vi "lv_icon.vi"(10 "Color icon in":T4={"image type"=0, "image depth"=8, "image"=[255, 255, 255, 255, 255, 255, 255, 255, 255, 255, 255, 255, 255, 255, 255, 255, 255, 255, 255, 255, 255, 255, 255, 255, 255, 255, 255, 255, 255, 255, 255, 255, 255, 0, 0, 0, 0, 0, 0, 0, 0, 0, 0, 0, 0, 0, 0, 0, 0, 0, 0, 0, 0, 0, 0, 0, 0, 0, 0, 0, 0, 0, 0, 255, 255, 0, 0, 0, 0, 0, 0, 0, 0, 0, 0, 0, 0, 0, 0, 0, 0, 0, 0, 0, 0, 0, 0, 0, 0, 0, 0, 0, 0, 0, 0, 255, 255, 0, 0, 255, 255, 255, 255, 255, 255, 255, 255, 255, 255, 255, 255, 255, 255, 255, 255, 255, 255, 255, 0, 0, 0, 0, 0, 0, 0, 0, 0, 255, 255, 0, 0, 255, 250, 250, 250, 250, 250, 250, 250, 250, 250, 250, 250, 250, 248, 250, 44, 250, 44, 255, 0, 0, 0, 0, 0, 0, 0, 0, 0, 255, 255, 0, 0, 255, 250, 255, 255, 255, 255, 255, 255, 255, 255, 255, 255, 255, 248, 250, 44, 250, 44, 255, 0, 0, 0, 0, 0, 0, 0, 0, 0, 255, 255, 0, 0, 255, 250, 255, 209, 197, 209, 255, 255, 255, 209, 197, 209, 255, 248, 252, 43, 252, 44, 255, 0, 0, 0, 0, 0, 0, 0, 0, 0, 255, 255, 0, 0, 255, 250, 255, 197, 255, 197, 255, 255, 255, 197, 255, 197, 255, 248, 44, 44, 44, 44, 255, 0, 0, 0, 0, 0, 0, 0, 0, 0, 255, 255, 0, 0, 255, 250, 209, 197, 255, 197, 209, 255, 209, 197, 255, 197, 209, 248, 43, 252, 43, 44, 255, 0, 0, 0, 0, 0, 0, 0, 0, 0, 255, 255, 0, 0, 255, 250, 197, 209, 255, 209, 197, 255, 197, 209, 255, 209, 197, 248, 252, 8, 252, 44, 255, 0, 0, 0, 0, 0, 0, 0, 0, 0, 255, 255, 0, 0, 255, 250, 197, 255, 255, 255, 197, 255, 197, 255, 255, 255, 197, 248, 252, 8, 252, 44, 255, 0, 0, 0, 0, 0, 0, 0, 0, 0, 255, 255, 0, 0, 255, 250, 255, 255, 255, 255, 209, 197, 209, 255, 255, 255, 255, 248, 43, 252, 43, 44, 255, 0, 0, 0, 0, 0, 0, 0, 0, 0, 255, 255, 0, 0, 255, 250, 255, 255, 255, 255, 255, 255, 255, 255, 255, 255, 255, 248, 44, 44, 44, 44, 255, 0, 0, 0, 0, 0, 0, 0, 0, 0, 255, 255, 0, 0, 255, 248, 248, 248, 248, 248, 248, 248, 248, 248, 248, 248, 248, 248, 44, 44, 131, 131, 255, 0, 0, 0, 0, 0, 0, 0, 0, 0, 255, 255, 0, 0, 255, 44, 44, 44, 44, 44, 44, 44, 44, 44, 44, 44, 44, 44, 44, 44, 131, 5, 131, 131, 0, 0, 0, 0, 0, 0, 0, 0, 255, 255, 0, 0, 255, 44, 252, 44, 44, 44, 44, 44, 252, 44, 44, 44, 44, 35, 35, 35, 131, 5, 5, 5, 131, 131, 0, 0, 0, 0, 0, 0, 255, 255, 0, 0, 255, 252, 213, 252, 44, 44, 44, 252, 35, 252, 44, 35, 35, 44, 44, 44, 131, 5, 5, 255, 5, 5, 131, 131, 0, 0, 0, 0, 255, 255, 0, 0, 255, 44, 212, 44, 44, 44, 44, 35, 44, 44, 35, 44, 44, 44, 44, 44, 131, 5, 255, 255, 255, 5, 5, 5, 131, 35, 35, 0, 255, 255, 0, 0, 255, 255, 213, 255, 255, 255, 35, 255, 255, 35, 255, 255, 255, 255, 255, 255, 131, 5, 5, 255, 5, 5, 131, 131, 0, 0, 0, 0, 255, 255, 0, 0, 0, 0, 212, 0, 0, 0, 35, 0, 0, 35, 0, 0, 213, 212, 212, 213, 131, 5, 5, 5, 131, 131, 0, 0, 0, 0, 0, 0, 255, 255, 0, 0, 0, 0, 0, 213, 0, 0, 0, 35, 35, 0, 0, 212, 0, 0, 0, 0, 131, 5, 131, 131, 0, 0, 0, 0, 0, 0, 0, 0, 255, 255, 0, 0, 0, 0, 0, 0, 212, 212, 0, 0, 0, 0, 213, 0, 0, 0, 0, 0, 131, 131, 0, 0, 0, 0, 0, 0, 0, 0, 0, 0, 255, 255, 0, 0, 0, 0, 0, 0, 0, 0, 213, 212, 213, 212, 0, 0, 0, 0, 0, 0, 0, 0, 0, 0, 0, 0, 255, 255, 0, 0, 0, 0, 255, 255, 0, 0, 0, 0, 0, 0, 0, 0, 0, 0, 0, 0, 0, 0, 0, 0, 0, 0, 0, 0, 0, 0, 0, 255, 0, 0, 255, 0, 0, 0, 255, 255, 0, 0, 0, 0, 0, 0, 0, 0, 0, 0, 0, 0, 0, 0, 0, 0, 0, 0, 0, 0, 0, 0, 0, 0, 0, 0, 255, 0, 0, 0, 255, 255, 0, 0, 0, 0, 0, 0, 0, 0, 0, 0, 0, 0, 0, 0, 0, 0, 0, 0, 0, 0, 0, 0, 0, 0, 255, 255, 0, 0, 0, 0, 255, 255, 0, 0, 0, 0, 0, 0, 0, 0, 0, 0, 0, 0, 0, 0, 0, 0, 0, 0, 0, 0, 0, 0, 0, 0, 0, 0, 255, 0, 0, 0, 255, 255, 0, 0, 0, 0, 0, 0, 0, 0, 0, 0, 0, 0, 0, 0, 0, 0, 0, 0, 0, 0, 0, 0, 0, 255, 0, 0, 255, 0, 0, 0, 255, 255, 0, 0, 0, 0, 0, 0, 0, 0, 0, 0, 0, 0, 0, 0, 0, 0, 0, 0, 0, 0, 0, 0, 0, 0, 255, 255, 0, 0, 0, 0, 255, 255, 0, 0, 0, 0, 0, 0, 0, 0, 0, 0, 0, 0, 0, 0, 0, 0, 0, 0, 0, 0, 0, 0, 0, 0, 0, 0, 0, 0, 0, 0, 255, 255, 0, 0, 0, 0, 0, 0, 0, 0, 0, 0, 0, 0, 0, 0, 0, 0, 0, 0, 0, 0, 0, 0, 0, 0, 0, 0, 0, 0, 0, 0, 255, 255, 255, 255, 255, 255, 255, 255, 255, 255, 255, 255, 255, 255, 255, 255, 255, 255, 255, 255, 255, 255, 255, 255, 255, 255, 255, 255, 255, 255, 255, 255, 255], "mask"=[], "colors"=[16777215, 16777164, 16777113, 16777062, 16777011, 16776960, 16764159, 16764108, 16764057, 16764006, 16763955, 16763904, 16751103, 16751052, 16751001, 16750950, 16750899, 16750848, 16738047, 16737996, 16737945, 16737894, 16737843, 16737792, 16724991, 16724940, 16724889, 16724838, 16724787, 16724736, 16711935, 16711884, 16711833, 16711782, 16711731, 16711680, 13434879, 13434828, 13434777, 13434726, 13434675, 13434624, 13421823, 13421772, 13421721, 13421670, 13421619, 13421568, 13408767, 13408716, 13408665, 13408614, 13408563, 13408512, 13395711, 13395660, 13395609, 13395558, 13395507, 13395456, 13382655, 13382604, 13382553, 13382502, 13382451, 13382400, 13369599, 13369548, 13369497, 13369446, 13369395, 13369344, 10092543, 10092492, 10092441, 10092390, 10092339, 10092288, 10079487, 10079436, 10079385, 10079334, 10079283, 10079232, 10066431, 10066380, 10066329, 10066278, 10066227, 10066176, 10053375, 10053324, 10053273, 10053222, 10053171, 10053120, 10040319, 10040268, 10040217, 10040166, 10040115, 10040064, 10027263, 10027212, 10027161, 10027110, 10027059, 10027008, 6750207, 6750156, 6750105, 6750054, 6750003, 6749952, 6737151, 6737100, 6737049, 6736998, 6736947, 6736896, 6724095, 6724044, 6723993, 6723942, 6723891, 6723840, 6711039, 6710988, 6710937, 6710886, 6710835, 6710784, 6697983, 6697932, 6697881, 6697830, 6697779, 6697728, 6684927, 6684876, 6684825, 6684774, 6684723, 6684672, 3407871, 3407820, 3407769, 3407718, 3407667, 3407616, 3394815, 3394764, 3394713, 3394662, 3394611, 3394560, 3381759, 3381708, 3381657, 3381606, 3381555, 3381504, 3368703, 3368652, 3368601, 3368550, 3368499, 3368448, 3355647, 3355596, 3355545, 3355494, 3355443, 3355392, 3342591, 3342540, 3342489, 3342438, 3342387, 3342336, 65535, 65484, 65433, 65382, 65331, 65280, 52479, 52428, 52377, 52326, 52275, 52224, 39423, 39372, 39321, 39270, 39219, 39168, 26367, 26316, 26265, 26214, 26163, 26112, 13311, 13260, 13209, 13158, 13107, 13056, 255, 204, 153, 102, 51, 15597568, 14483456, 12255232, 11141120, 8912896, 7798784, 5570560, 4456448, 2228224, 1114112, 60928, 56576, 47872, 43520, 34816, 30464, 21760, 17408, 8704, 4352, 238, 221, 187, 170, 136, 119, 85, 68, 34, 17, 15658734, 14540253, 12303291, 11184810, 8947848, 7829367, 5592405, 4473924, 2236962, 1118481, 0], "Rectangle"={"left"=0, "top"=0, "right"=32, "bottom"=32}}, 11 "BW icon in":T4={"image type"=0, "image depth"=1, "image"=[255, 255, 255, 255, 128, 0, 0, 1, 128, 0, 0, 1, 159, 255, 252, 1, 144, 0, 84, 1, 151, 255, 84, 1, 150, 251, 84, 1, 149, 117, 4, 1, 149, 117, 36, 1, 147, 174, 84, 1, 147, 174, 84, 1, 151, 223, 36, 1, 151, 255, 4, 1, 144, 0, 28, 1, 144, 0, 22, 1, 148, 16, 241, 129, 158, 59, 18, 97, 148, 36, 23, 29, 159, 255, 242, 97, 132, 73, 241, 129, 130, 50, 22, 1, 129, 132, 24, 1, 128, 120, 0, 97, 128, 0, 0, 145, 128, 0, 0, 17, 128, 0, 0, 97, 128, 0, 0, 17, 128, 0, 0, 145, 128, 0, 0, 97, 128, 0, 0, 1, 128, 0, 0, 1, 255, 255, 255, 255], "mask"=[], "colors"=[16777215, 0], "Rectangle"={"left"=0, "top"=0, "right"=32, "bottom"=32}}) -> (0 "Error code out":i32=43, 2 "Color icon out":T4={"image type"=0, "image depth"=24, "image"=array[3072 elements], "mask"=[0, 0, 0, 0, 0, 0, 0, 0, 0, 0, 0, 0, 0, 0, 0, 0, 0, 0, 0, 0, 0, 0, 0, 0, 0, 0, 0, 0, 0, 0, 0, 0, 0, 0, 0, 0, 0, 0, 0, 0, 0, 0, 0, 0, 0, 0, 0, 0, 0, 0, 0, 0, 0, 0, 0, 0, 0, 0, 0, 0, 0, 0, 0, 0, 0, 0, 0, 0, 0, 0, 0, 0, 0, 0, 0, 0, 0, 0, 0, 0, 0, 0, 0, 0, 0, 0, 0, 0, 0, 0, 0, 0, 0, 0, 0, 0, 0, 0, 0, 0, 0, 0, 0, 0, 0, 0, 0, 0, 0, 0, 0, 0, 0, 0, 0, 0, 0, 0, 0, 0, 0, 0, 0, 0, 0, 0, 0, 0], "colors"=[], "Rectangle"={"left"=0, "top"=0, "right"=32, "bottom"=32}}, 3 "BW icon out":T4={"image type"=0, "image depth"=1, "image"=[0, 0, 0, 0, 0, 0, 0, 0, 0, 0, 0, 0, 0, 0, 0, 0, 0, 0, 0, 0, 0, 0, 0, 0, 0, 0, 0, 0, 0, 0, 0, 0, 0, 0, 0, 0, 0, 0, 0, 0, 0, 0, 0, 0, 0, 0, 0, 0, 0, 0, 0, 0, 0, 0, 0, 0, 0, 0, 0, 0, 0, 0, 0, 0, 0, 0, 0, 0, 0, 0, 0, 0, 0, 0, 0, 0, 0, 0, 0, 0, 0, 0, 0, 0, 0, 0, 0, 0, 0, 0, 0, 0, 0, 0, 0, 0, 0, 0, 0, 0, 0, 0, 0, 0, 0, 0, 0, 0, 0, 0, 0, 0, 0, 0, 0, 0, 0, 0, 0, 0, 0, 0, 0, 0, 0, 0, 0, 0], "mask"=[], "colors"=[16777215, 0], "Rectangle"={"left"=0, "top"=0, "right"=32, "bottom"=32}})   [LabVIEW 2021, in "lv_icon.lvlib"]
doc: "<p>Display this dialog box in one of the following ways:</p>\n\n<ul>\n<li>Double-click the <a href=\"nihelplauncher://docs/csh?context=lvcore_lvconcepts_using_icons\">icon</a> in the upper right corner of the front panel window, block diagram window, or <a href=\"nihelplauncher://docs/csh?context=lvcore_lvconcepts_custom_cont_ind_type\">Control Editor</a> window.</li>\n<li>Right-click the icon in the upper right corner of the front panel window, block diagram window, or <strong>Control Editor</strong> window and select <strong>Edit Icon</strong> from the shortcut menu.</li>\n<li>Select <strong>File<span class=\"U+187\">>></span>VI Properties</strong> or <strong>File<span class=\"U+187\">>></span>Control Properties</strong> to display the <a href=\"nihelplauncher://docs/csh?context=lvcore_lvdialog_vi_properties_dialog_box\">VI Properties</a> dialog box or <strong>Control Properties</strong> dialog box, respectively. Then select <strong>General</strong> from the <strong>Category</strong> pull-down menu and click the <strong>Edit Icon</strong> button.</li>\n<li>Right-click a project library, statechart, class, or XControl item in the <a href=\"nihelplauncher://docs/csh?context=lvcore_lvconcepts_using_labview_projects\">Project Explorer</a> window and select <strong> Properties</strong> from the shortcut menu to display the corresponding <strong>Properties</strong> dialog box. Then click the <strong>Edit</strong> button on the <strong>General Settings</strong> page.</li>\n</ul>\n\n<p>Use this dialog box to <a href=\"nihelplauncher://docs/csh?context=lvcore_lvhowto_creating_icons\">create and edit icons</a>.</p>"
uses:
  <vilib>/LabVIEW Icon API/lv_icon/lv_icon.lvlib
  <vilib>/LabVIEW Icon API/lv_icon/Controls/BodyText.ctl
  <vilib>/LabVIEW Icon API/lv_icon/Controls/Font.ctl
  <vilib>/LabVIEW Icon API/lv_icon/Controls/Alignment.ctl
  <vilib>/LabVIEW Icon API/lv_icon/Controls/Layer.ctl
  <resource>/plugins/NIIconEditor/Controls/LayerList.ctl
  <resource>/plugins/NIIconEditor/Controls/NewLayer.ctl
  <resource>/plugins/NIIconEditor/Controls/DeleteLayer.ctl
  <resource>/plugins/NIIconEditor/Controls/Arrow Up.ctl
  <resource>/plugins/NIIconEditor/Controls/Arrow Down.ctl
  <resource>/plugins/NIIconEditor/Controls/Framework Templates.ctl
  <vilib>/LabVIEW Icon API/lv_icon/Controls/Graphic.ctl
  <resource>/plugins/NIIconEditor/Controls/ColorChange.ctl
  <vilib>/LabVIEW Icon API/lv_icon/Controls/IEColor.ctl
  <resource>/plugins/NIIconEditor/Controls/Rotate.ctl
  <resource>/plugins/NIIconEditor/Controls/Flip.ctl
  <resource>/plugins/NIIconEditor/Controls/Tools.ctl
  <resource>/plugins/NIIconEditor/Controls/Pen.ctl
  <resource>/plugins/NIIconEditor/Controls/Line.ctl
  <resource>/plugins/NIIconEditor/Controls/Dropper.ctl
  <resource>/plugins/NIIconEditor/Controls/Fill.ctl
  <resource>/plugins/NIIconEditor/Controls/IERect.ctl
  <resource>/plugins/NIIconEditor/Controls/FRect.ctl
  <resource>/plugins/NIIconEditor/Controls/Circle.ctl
  <resource>/plugins/NIIconEditor/Controls/FCircle.ctl
  <resource>/plugins/NIIconEditor/Controls/Rubber.ctl
  <resource>/plugins/NIIconEditor/Controls/Text.ctl
  <resource>/plugins/NIIconEditor/Controls/Selection.ctl
  <resource>/plugins/NIIconEditor/Controls/Move.ctl
  <resource>/plugins/NIIconEditor/Controls/TextMarker.ctl
  <vilib>/picture/picture.llb/imagedata.ctl
  <resource>/plugins/NIIconEditor/Controls/Path&Icon.ctl
  <resource>/plugins/NIIconEditor/Controls/Refresh.ctl
  <vilib>/Utility/miscctls.llb/LVKeyNavTypeDef.ctl
  <resource>/plugins/NIIconEditor/Controls/References Cluster.ctl
  <vilib>/Utility/miscctls.llb/LVPoint32TypeDef.ctl
  <vilib>/LabVIEW Icon API/lv_icon/Controls/Pathes.ctl
  <resource>/plugins/NIIconEditor/Class/Ants/Ants.lvclass
  <resource>/plugins/NIIconEditor/Class/FakedArray/FakedArray.lvclass
  <vilib>/LabVIEW Icon API/lv_icon/Classes/Icon/Icon.lvclass
  <resource>/plugins/NIIconEditor/Class/Icon Library/Glyph.lvclass
  <resource>/dialog/lvconfig.llb/LV Config Read String.vi
  <resource>/dialog/lvconfig.llb/LV Config Write String.vi
panel:
  out "LabVIEW Icon out":string
  in  "LabVIEW Icon in":string
  out "Terminals":picture
  out "Preview2":picture
  in  "?":cluster{T1[], i32, bool}
  out "TextMarker":T2="^"
  in  "Help":bool
  in  "Cancel":bool
  in  "OK":bool
  out "XYZ":string="X: 14\nY: 31\nZ: 1"
  out "RGB":string="R: 0\nG: 0\nB: 0"
  out "Icon":picture
  out "Clipboard":picture
  in  "?":T3[](array[typedef])
  in  "Tab Control":T5(tab)
  in  "refreshTemplates":T6
  out "templates path str":string
  in  "Templates":string(tree)="<All>"
  in  "Filter templates by keyword":string
  in  "Framework Templates":T7={"Scrollbar"=0, "Path & Icon 1"={"Rectangle"={"left"=0, "top"=0, "right"=32, "bottom"=32}, "Path"=path "C:/Users/tsandris/Documents/LabVIEW Data/Icon Templates/VI/Frameworks/_blank.png", "Image"=bytes[3230], "Filter"="VI\\Frameworks", "FileName"="_blank"}, "Path & Icon 2"={"Rectangle"={"left"=0, "top"=0, "right"=32, "bottom"=32}, "Path"=path "C:/Users/tsandris/Documents/LabVIEW Data/Icon Templates/Library/Frameworks/_blank.png", "Image"=bytes[3230], "Filter"="Library\\Frameworks", "FileName"="_blank"}, "Path & Icon 3"={"Rectangle"={"left"=0, "top"=0, "right"=0, "bottom"=0}, "Path"=path "", "Image"=bytes[0], "Filter"="", "FileName"=""}, "Path & Icon 4"={"Rectangle"={"left"=0, "top"=0, "right"=0, "bottom"=0}, "Path"=path "", "Image"=bytes[0], "Filter"="", "FileName"=""}, "Path & Icon 5"={"Rectangle"={"left"=0, "top"=0, "right"=0, "bottom"=0}, "Path"=path "", "Image"=bytes[0], "Filter"="", "FileName"=""}, "Path & Icon 6"={"Rectangle"={"left"=0, "top"=0, "right"=0, "bottom"=0}, "Path"=path "", "Image"=bytes[0], "Filter"="", "FileName"=""}, "Path & Icon 7"={"Rectangle"={"left"=0, "top"=0, "right"=0, "bottom"=0}, "Path"=path "", "Image"=bytes[0], "Filter"="", "FileName"=""}, "Path & Icon 8"={"Rectangle"={"left"=0, "top"=0, "right"=0, "bottom"=0}, "Path"=path "", "Image"=bytes[0], "Filter"="", "FileName"=""}, "Path & Icon 9"={"Rectangle"={"left"=0, "top"=0, "right"=0, "bottom"=0}, "Path"=path "", "Image"=bytes[0], "Filter"="", "FileName"=""}, "Path & Icon 10"={"Rectangle"={"left"=0, "top"=0, "right"=0, "bottom"=0}, "Path"=path "", "Image"=bytes[0], "Filter"="", "FileName"=""}, "Path & Icon 11"={"Rectangle"={"left"=0, "top"=0, "right"=0, "bottom"=0}, "Path"=path "", "Image"=bytes[0], "Filter"="", "FileName"=""}, "Path & Icon 12"={"Rectangle"={"left"=0, "top"=0, "right"=0, "bottom"=0}, "Path"=path "", "Image"=bytes[0], "Filter"="", "FileName"=""}, "Path & Icon 13"={"Rectangle"={"left"=0, "top"=0, "right"=0, "bottom"=0}, "Path"=path "", "Image"=bytes[0], "Filter"="", "FileName"=""}, "Path & Icon 14"={"Rectangle"={"left"=0, "top"=0, "right"=0, "bottom"=0}, "Path"=path "", "Image"=bytes[0], "Filter"="", "FileName"=""}, "Path & Icon 15"={"Rectangle"={"left"=0, "top"=0, "right"=0, "bottom"=0}, "Path"=path "", "Image"=bytes[0], "Filter"="", "FileName"=""}, "Path & Icon 16"={"Rectangle"={"left"=0, "top"=0, "right"=0, "bottom"=0}, "Path"=path "", "Image"=bytes[0], "Filter"="", "FileName"=""}, "Path & Icon 17"={"Rectangle"={"left"=0, "top"=0, "right"=0, "bottom"=0}, "Path"=path "", "Image"=bytes[0], "Filter"="", "FileName"=""}, "Path & Icon 18"={"Rectangle"={"left"=0, "top"=0, "right"=0, "bottom"=0}, "Path"=path "", "Image"=bytes[0], "Filter"="", "FileName"=""}, "Path & Icon 19"={"Rectangle"={"left"=0, "top"=0, "right"=0, "bottom"=0}, "Path"=path "", "Image"=bytes[0], "Filter"="", "FileName"=""}, "Path & Icon 20"={"Rectangle"={"left"=0, "top"=0, "right"=0, "bottom"=0}, "Path"=path "", "Image"=bytes[0], "Filter"="", "FileName"=""}, "Path & Icon 21"={"Rectangle"={"left"=0, "top"=0, "right"=0, "bottom"=0}, "Path"=path "", "Image"=bytes[0], "Filter"="", "FileName"=""}, "Path & Icon 22"={"Rectangle"={"left"=0, "top"=0, "right"=0, "bottom"=0}, "Path"=path "", "Image"=bytes[0], "Filter"="", "FileName"=""}, "Path & Icon 23"={"Rectangle"={"left"=0, "top"=0, "right"=0, "bottom"=0}, "Path"=path "", "Image"=bytes[0], "Filter"="", "FileName"=""}, "Path & Icon 24"={"Rectangle"={"left"=0, "top"=0, "right"=0, "bottom"=0}, "Path"=path "", "Image"=bytes[0], "Filter"="", "FileName"=""}, "Path & Icon 25"={"Rectangle"={"left"=0, "top"=0, "right"=0, "bottom"=0}, "Path"=path "", "Image"=bytes[0], "Filter"="", "FileName"=""}, "Path & Icon 26"={"Rectangle"={"left"=0, "top"=0, "right"=0, "bottom"=0}, "Path"=path "", "Image"=bytes[0], "Filter"="", "FileName"=""}, "Path & Icon 27"={"Rectangle"={"left"=0, "top"=0, "right"=0, "bottom"=0}, "Path"=path "", "Image"=bytes[0], "Filter"="", "FileName"=""}, "Path & Icon 28"={"Rectangle"={"left"=0, "top"=0, "right"=0, "bottom"=0}, "Path"=path "", "Image"=bytes[0], "Filter"="", "FileName"=""}, "Path & Icon 29"={"Rectangle"={"left"=0, "top"=0, "right"=0, "bottom"=0}, "Path"=path "", "Image"=bytes[0], "Filter"="", "FileName"=""}, "Path & Icon 30"={"Rectangle"={"left"=0, "top"=0, "right"=0, "bottom"=0}, "Path"=path "", "Image"=bytes[0], "Filter"="", "FileName"=""}}
  out "Class path":path
  in  "Action":string
  in  "Execute custom override":bool
  in  "Use PPL":bool=TRUE
  in  "Body Text":T8={"Line 1 text"="", "Line 2 text"="", "Line 3 text"="", "Line 4 text"="", "Line 1 color"=0, "Line 2 color"=0, "Line 3 color"=0, "Line 4 color"=0, "Body Text Spec"={"Font"="", "Alignment"=1, "Size"=9}, "Center text vertically"=TRUE, "Capitalize Text"=TRUE} {"Body Text Spec"."Alignment" items=["left", "center", "right"]}
  in  "Filter glyphs by keyword":string
  in  "Glyphs":string(tree)="<All>"
  out "glyph path str":string
  out "Glyphs []":T1[][](array[typedef])
  in  "refreshGlyphs":T6
  in  "Add Layer":T11
  in  "Remove Layer":T12
  in  "Move Down":T13
  in  "Move Up":T14
  in  "Icon Template":T15={"LayerIcon"=bytes[0], "LayerName"="", "Opacity"=100, "Visibility?"=TRUE} {"Opacity" scale=0.0..100.0}
  in  "Icon Text":T15={"LayerIcon"=bytes[0], "LayerName"="Icon Text", "Opacity"=100, "Visibility?"=TRUE} {"Opacity" scale=0.0..100.0}
  in  "User Layers":T16={"Scrollbar"=0, "Layer 1"={"LayerIcon"=bytes[3230], "LayerName"="VI Icon", "Opacity"=100, "Visibility?"=TRUE}, "Layer 2"={"LayerIcon"=bytes[3230], "LayerName"="", "Opacity"=100, "Visibility?"=TRUE}, "Layer 3"={"LayerIcon"=bytes[3230], "LayerName"="", "Opacity"=100, "Visibility?"=TRUE}, "Layer 4"={"LayerIcon"=bytes[3230], "LayerName"="", "Opacity"=100, "Visibility?"=TRUE}} {"Layer 4"."Opacity" scale=0.0..100.0; "Layer 3"."Opacity" scale=0.0..100.0; "Layer 2"."Opacity" scale=0.0..100.0; "Layer 1"."Opacity" scale=0.0..100.0}
  out "Preview":picture
  in  "Horizontal Flip":T17
  in  "Clockwise Rotate":T18
  in  "Swap":T19
  in  "Line Color":T20
  in  "Fill Color":T20=16777215
  in  "Tools":T21=enum."Rectangle"
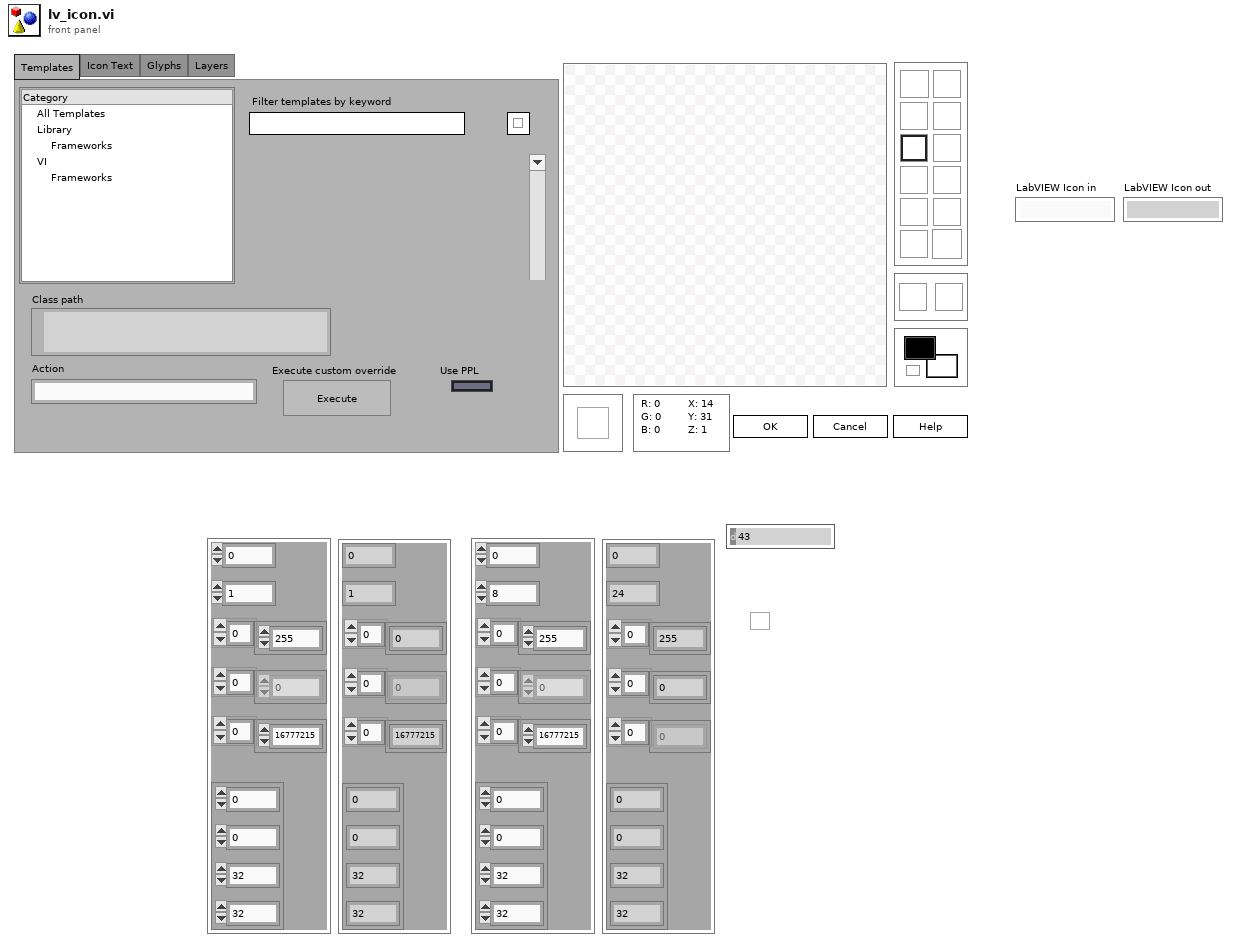
[diagram p1: front panel]
types:
  T1 = typedef "Graphic.ctl" = cluster{"Rectangle":cluster{"left":i16, "top":i16, "right":i16, "bottom":i16}, "Path":path, "Image":picture, "Filter":string, "FileName":string}
  T2 = typedef "TextMarker.ctl" = string
  T3 = typedef "Path&Icon.ctl" = cluster{"Rectangle":cluster{"left":i16, "top":i16, "right":i16, "bottom":i16}, "Path":path, "Image":picture, "Filter":string, "FileName":string}
  T4 = typedef "imagedata.ctl" = cluster{"image type":i32, "image depth":i32, "image":u8[], "mask":u8[], "colors":u32[], "Rectangle":cluster{"left":i16, "top":i16, "right":i16, "bottom":i16}}
  T5 = enum32{"Templates", "Icon Text", "Glyphs", "Layers"}
  T6 = typedef "Refresh.ctl" = bool
  T7 = typedef "Framework Templates.ctl" = cluster{"Scrollbar":i32, "Path & Icon 1":T1, "Path & Icon 2":T1, "Path & Icon 3":T1, "Path & Icon 4":T1, "Path & Icon 5":T1, "Path & Icon 6":T1, "Path & Icon 7":T1, "Path & Icon 8":T1, "Path & Icon 9":T1, "Path & Icon 10":T1, "Path & Icon 11":T1, "Path & Icon 12":T1, "Path & Icon 13":T1, "Path & Icon 14":T1, "Path & Icon 15":T1, "Path & Icon 16":T1, "Path & Icon 17":T1, "Path & Icon 18":T1, "Path & Icon 19":T1, "Path & Icon 20":T1, "Path & Icon 21":T1, "Path & Icon 22":T1, "Path & Icon 23":T1, "Path & Icon 24":T1, "Path & Icon 25":T1, "Path & Icon 26":T1, "Path & Icon 27":T1, "Path & Icon 28":T1, "Path & Icon 29":T1, "Path & Icon 30":T1}
  T8 = typedef "BodyText.ctl" = cluster{"Line 1 text":string, "Line 2 text":string, "Line 3 text":string, "Line 4 text":string, "Line 1 color":u32, "Line 2 color":u32, "Line 3 color":u32, "Line 4 color":u32, "Body Text Spec":cluster{"Font":T9, "Alignment":T10, "Size":u8}, "Center text vertically":bool, "Capitalize Text":bool}
  T9 = typedef "Font.ctl" = string
  T10 = typedef "Alignment.ctl" = u16
  T11 = typedef "NewLayer.ctl" = bool
  T12 = typedef "DeleteLayer.ctl" = bool
  T13 = typedef "Arrow Down.ctl" = bool
  T14 = typedef "Arrow Up.ctl" = bool
  T15 = typedef "Layer.ctl" = cluster{"LayerIcon":picture, "LayerName":string, "Opacity":u8, "Visibility?":bool}
  T16 = typedef "LayerList.ctl" = cluster{"Scrollbar":i32, "Layer 1":T15, "Layer 2":T15, "Layer 3":T15, "Layer 4":T15}
  T17 = typedef "Flip.ctl" = bool
  T18 = typedef "Rotate.ctl" = bool
  T19 = typedef "ColorChange.ctl" = bool
  T20 = typedef "IEColor.ctl" = u32
  T21 = typedef "Tools.ctl" = enum32{"Pencil", "Line", "Dropper", "Fill", "Rectangle", "Filled Rectangle", "Ellipse", "Filled Ellipse", "Eraser", "Text", "Select", "Move"}
  T22 = enum32{"Invalid", "Standard", "Closed", "Hidden", "Minimized", "Maximized"}
  T23 = typedef "References Cluster.ctl" = cluster{"Add Layer":refnum<vi>, "Remove Layer":refnum<vi>, "Line Text":refnum<vi>[], "Body Text Spec":refnum<vi>, "DNL_Font":refnum<vi>, "glyph path str":refnum<vi>, "templates path str":refnum<vi>, "Arrow Up":refnum<vi>, "Arrow Down":refnum<vi>, "IE VI Ref":refnum<vi>, "Glyphs tree":refnum<vi>, "Templates tree":refnum<vi>, "Layer Icon Text":refnum<vi>, "Layer Template":refnum<vi>, "Clipboard":refnum<vi>, "BW icon in":refnum<vi>, "Color icon in":refnum<vi>, "Layer Clust":refnum<vi>, "Body Text":refnum<vi>, "DNL_Framework Templates":refnum<vi>, "Search Templates":refnum<vi>, "TextMarker":refnum<vi>, "Tab Control":refnum<vi>, "Search Glyphs":refnum<vi>, "Line Color":refnum<vi>, "DNL_Glyphs []":refnum<vi>, "Fill Color":refnum<vi>, "Tools":refnum<vi>, "Glyphs tree":refnum<vi>, "Icon":refnum<vi>, "Preview":refnum<vi>, "Ants":refnum<vi>, "Terminals":refnum<vi>, "menu reference":refnum<k9>, "LayerNames":refnum<vi>[], "GlyphLoadAnimation":refnum<vi>, "TemplateLoadAnimation":refnum<vi>, "refreshGlyphs":refnum<vi>, "refreshTemplates":refnum<vi>}
  T24 = typedef "LVKeyNavTypeDef.ctl" = cluster{"Control":bool, "Shift":bool, "Key":string}
  T25 = cluster{"Left":i16, "Top":i16, "Right":i16, "Bottom":i16}
  T26 = typedef "LVAllMonitorsDisplayTypeDef.ctl" = cluster{"Bounds":cluster{"Left":i16, "Top":i16, "Right":i16, "Bottom":i16}, "Depth":i16}[]
  T27 = cluster{"Global stop?":refnum<user-event>, "Templates":refnum<user-event>, "Glyphs":refnum<user-event>}
  T28 = typedef "IE Data.ctl" = cluster{"Class":T29, "Ref":T23, "Support":T30}
  T29 = typedef "IE Classes.ctl" = cluster{"Ants":refnum<class "Ants.lvclass">, "Layer":refnum<class "FakedArray.lvclass">, "Templates":refnum<class "FakedArray.lvclass">, "Icon":refnum<class "Icon.lvclass">, "Glyph":refnum<class "Glyph.lvclass">, "Settings":refnum<class "Settings.lvclass">, "Tools":refnum<class "Tools Paint.lvclass">}
  T30 = typedef "SupportClass.ctl" = cluster{"AntsRect":cluster{"left":i16, "top":i16, "right":i16, "bottom":i16}, "Mouse Move Coords":T31, "Mouse Down Coords":T31, "Temp Coord":T31, "Action":T32, "Edge Color":T20, "Fill Color":T20, "Mouse Down?":bool, "Draft Mode?":bool, "Temp Icon":picture, "CTRL Pressed":bool, "Move Selection?":bool, "AntsRect Orig":cluster{"left":i16, "top":i16, "right":i16, "bottom":i16}, "Text":string, "TM Set?":bool, "Mouse inside icon?":bool, "Tool (old value)":u32, "Pencil Move Color":u32, "Swap Colors?":bool, "Shift pressed?":bool}
  T31 = typedef "LVPoint32TypeDef.ctl" = cluster{"Horizontal":i32, "Vertical":i32}
  T32 = typedef "SupportClass_Action.ctl" = enum16{"Default", "Move Selection", "Glyph Library", "Tool"}
  T33 = typedef "Pathes.ctl" = enum16{"Root Path", "Icon Templates", "Icon Templates VI", "Icon Templates Lib", "Glyphs"}
  T34 = typedef "lveventtype.ctl" = enum32{"Null", "Timeout", "Annotation Menu Selection", "Annotation Menu Selection?", "App Instance Close", "App Instance Close?", "Autoscale Range Change", "Bookmark Info Change", "Cell Edit", "Cell Edit?", "Cursor Grab", "Cursor Grab?", "Cursor Menu Selection", "Cursor Menu Selection?", "Cursor Move", "Cursor Release", "Data Change", "Direction Change", "Display State Change", "Drag Ended", "Drag Enter", "Drag Leave", "Drag Over", "Drag Source Update", "Drag Starting", "Drag Starting?", "Drop", "Exec State Change", "Key Down", "Key Down?", "Key Repeat", "Key Repeat?", "Key Up", "Listbox Double Click", "Menu Activation?", "Menu Selection (App)", "Menu Selection? (App)", "Menu Selection (User)", "Mouse Down", "Mouse Down?", "Mouse Enter", "Mouse Leave", "Mouse Move", "Mouse Up", "Mouse Wheel", "NI Security User Change (App)", "Pane Size", "Panel Close", "Panel Close?", "Panel Resize", "Plot Attribute Change", "Scale Range Change", "Shortcut Menu Activation?", "Shortcut Menu Selection (App)", "Shortcut Menu Selection? (App)", "Shortcut Menu Selection (User)", "Tree Double Click", "Tree Drag", "Tree Drag?", "Tree Drop", "Tree Drop?", "Tree Item Close", "Tree Item Close?", "Tree Item Open", "Tree Item Open?", "User Event", "Value Change"}
  T35 = typedef "eventvkey.ctl" = enum16{"ASCII", "Enter", "Return", "Shift", "Ctrl", "Alt", "Cmd", "Opt", "Caps", "NumLock", "Clear", "Break", "Up", "Down", "Left", "Right", "Insert", "Delete", "Home", "End", "PageUp", "PageDown", "Escape", "Help", "Pause", "ScrollLock", "F1", "F2", "F3", "F4", "F5", "F6", "F7", "F8", "F9", "F10", "F11", "F12", "F13", "F14", "F15", "F16", "F17", "F18", "F19", "F20", "F21", "F22", "F23", "F24", "Play", "VolumeUp", "VolumeDown", "Mute", "Two Byte Char"}
  T36 = cluster{"Shift":bool, "Ctrl":bool, "Alt":bool, "Cmd":bool, "Opt":bool}
  T37 = typedef "LVRectTypeDef.ctl" = cluster{"Left":i16, "Top":i16, "Right":i16, "Bottom":i16}
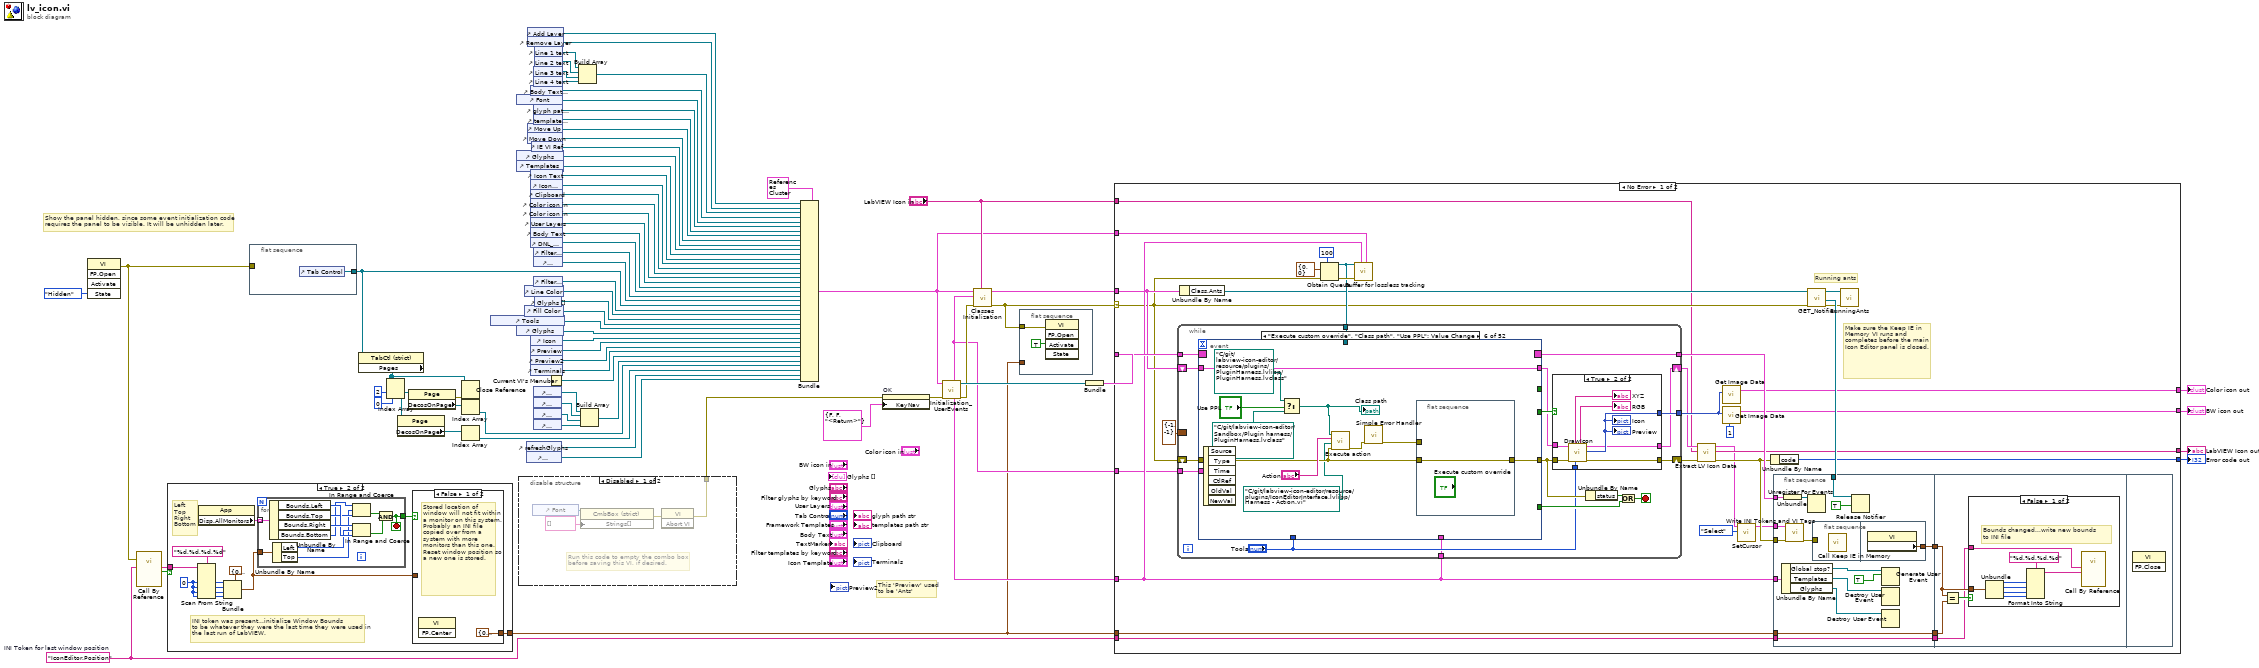
[diagram p0: block diagram]
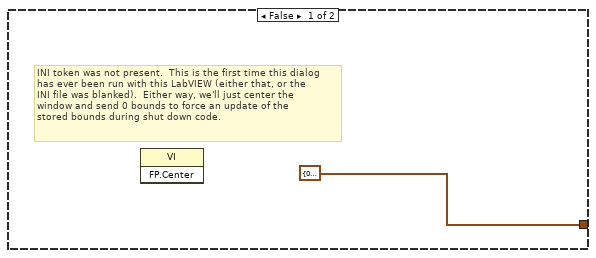
[diagram p2: hidden frame]
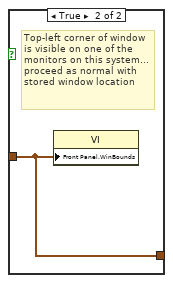
[diagram p3: hidden frame]
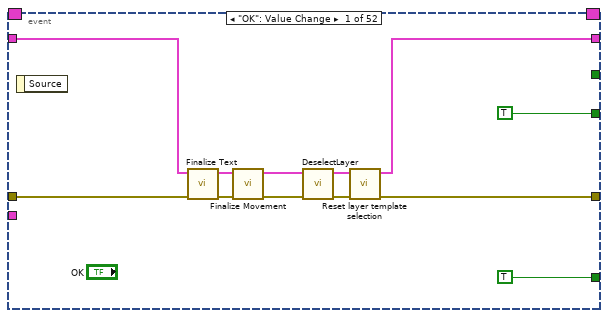
[diagram p6: hidden frame]
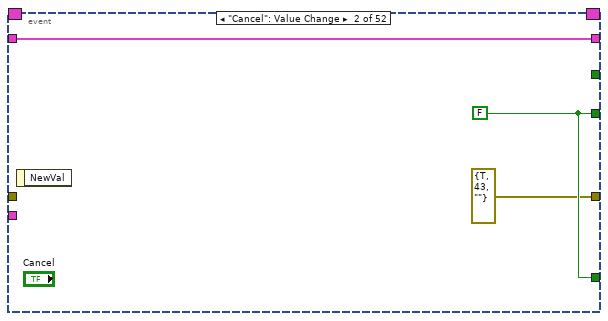
[diagram p7: hidden frame]
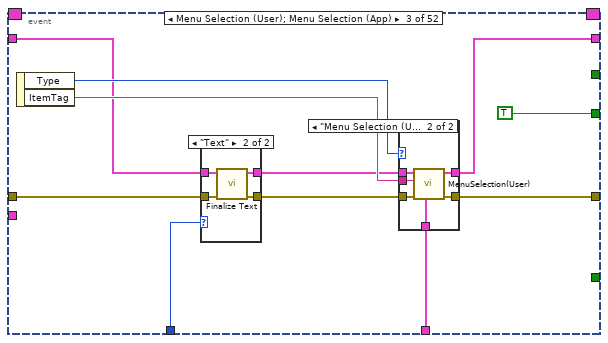
[diagram p8: hidden frame]
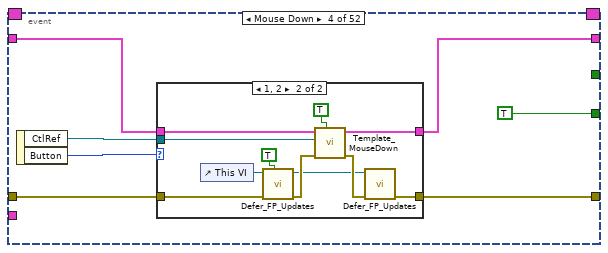
[diagram p11: hidden frame]
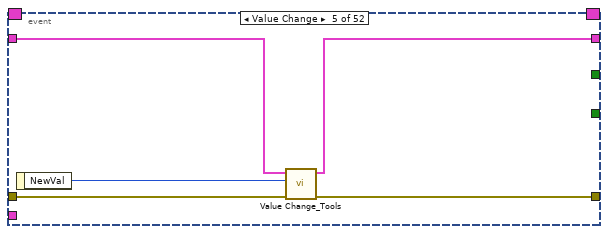
[diagram p13: hidden frame]
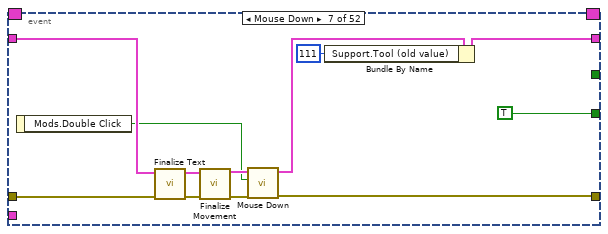
[diagram p14: hidden frame]
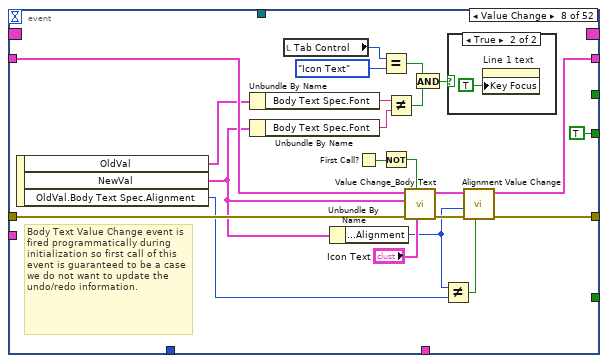
[diagram p15: hidden frame]
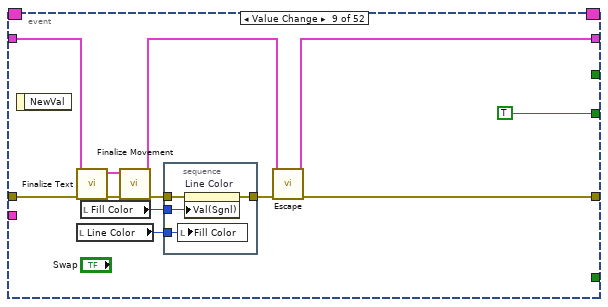
[diagram p17: hidden frame]
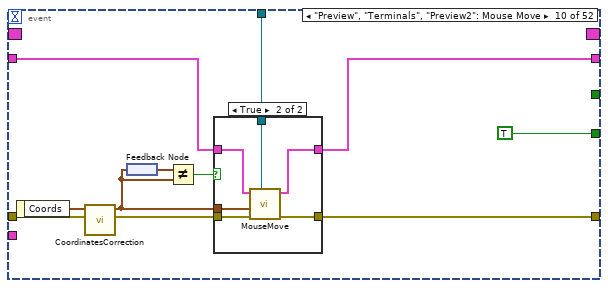
[diagram p18: hidden frame]
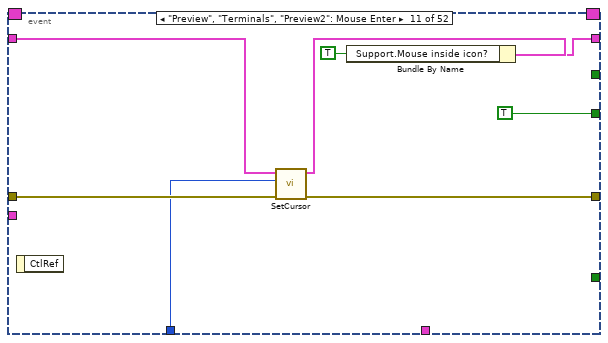
[diagram p20: hidden frame]
diagram:
  w1 = "IconEditor.Position"  # INI Token for last window position
  # "Show the panel hidden, since some event initialization code requires the panel to be visible. It will be unhidden later."
  # "This 'Preview' used\nto be 'Ants'"
  n1 = invoke class="VI" method="FP.Open"("State"=T22."Hidden") -> (error out=w3:errorcluster)  [unwired: 4 in, 4 out]
  n2 = call-by-ref "?"(error in=w3, "key"=w1) -> ("found?"=w4:bool, "value"=w5:string)  [unwired: 5 in, 3 out]
  n3 = case shown="True" w4 {
    tunnel: [T25 {"Left"=0, "Top"=0, "Right"=0, "Bottom"=0} ("Front Panel.PanelBounds") w79] -> w2
    tunnel: w5 -> [_ w90]
    frame False {
      # "INI token was not present.  This is the first time this dialog\nhas ever been run with this LabVIEW (either that, or the\nINI file was blanked).  Either way, we'll just center the\nwindow and send 0 bounds to force an update of the\nstored bounds during shut down code."
      n4 = invoke class="VI" method="FP.Center"() -> ()  [unwired: 3 in, 3 out]
    }
    frame True {
      w88 = i16 0 ("default value 1")
      # "Left\nTop\nRight\nBottom"
      # "INI token was present...initialize Window Bounds\nto be whatever they were the last time they were used in\nthe last run of LabVIEW."
      n5 = Scan From String(format string="%d,%d,%d,%d", input string=w90, default 1=w88, default 2=w88, default 3=w88, default 4=w88) -> (output 1=w87:i16, output 2=w86:i16, output 3=w85:i16, output 4=w84:i16)  [unwired: 2 in, 3 out]
      n6 = property class="App"() -> ("Disp.AllMonitors"=w82:T26)  [unwired: 2 in, 2 out]
      n7 = Bundle(cluster=T25 {"Left"=0, "Top"=0, "Right"=0, "Bottom"=0} ("Front Panel.PanelBounds"), "Left"=w87, "Top"=w86, "Right"=w85, "Bottom"=w84) -> (w81:T25)
      n8 = for {
        tunnel: w82 -> [w103] mode=indexing
        tunnel: w81 -> [w102]
        tunnel: [w93] -> w80
        stop <- w93 stop-if-true
        n9 = Unbundle By Name(w103) -> ("Bounds.Left"=w100:i16, "Bounds.Top"=w98:i16, "Bounds.Right"=w101:i16, "Bounds.Bottom"=w97:i16)
        n10 = Unbundle By Name(w102) -> ("Left"=w99:i16, "Top"=w96:i16)
        n11 = In Range and Coerce(upper limit=w97, x=w96, lower limit=w98) -> (In Range?=w95:bool)  [unwired: 1 out]
        n12 = In Range and Coerce(upper limit=w101, x=w99, lower limit=w100) -> (In Range?=w94:bool)  [unwired: 1 out]
        n13 = And(x=w95, y=w94) -> (x .and. y?=w93:bool)
      }
      n14 = case shown="False" w80 {
        tunnel: w81 -> [_ w92]
        tunnel: [T25 {"Left"=0, "Top"=0, "Right"=0, "Bottom"=0} ("Front Panel.PanelBounds") w92] -> w79
        frame False {
          # "Stored location of window will not fit within a monitor on this system.  Probably an INI file copied over from a system with more monitors than this one.  Reset window position so a new one is stored."
          n15 = invoke class="VI" method="FP.Center"() -> ()  [unwired: 3 in, 3 out]
        }
        frame True {
          # "Top-left corner of window is visible on one of the monitors on this system... proceed as normal with stored window location"
          n16 = property class="VI"("Front Panel.WinBounds"=w92) -> ()  [unwired: 2 in, 2 out]
        }
      }
    }
  }
  n17 = flat-sequence {
    tunnel: [w104] -> w18
    tunnel: w3 -> [_]
    frame #0 {
      n18 = control-ref of="Tab Control"() -> (w104:refnum<vi>)
    }
  }
  n19 = property class="TabCtl (strict)"(reference=w18) -> ("Pages"=w8:refnum<vi>[])  [unwired: 1 in, 2 out]
  n20 = Index Array(array=w8, index #1=2 ("index"), index #2=0 ("index")) -> (element #1=w14:refnum<vi>, element #2=w15:refnum<vi>)
  n21 = property class="Page"(reference=w15) -> ("DecosOnPage"=w12:refnum<vi>[])  [unwired: 1 in, 2 out]
  n22 = property class="Page"(reference=w14) -> (error out=w9:errorcluster, "DecosOnPage"=w13:refnum<vi>[])  [unwired: 1 in, 1 out]
  n23 = Close Reference(reference=w8, error in (no error)=w9) -> ()  [unwired: 1 out]
  n24 = Index Array(array=w13) -> (element=w10:refnum<vi>)  [unwired: 1 in]
  n25 = Index Array(array=w12) -> (element=w11:refnum<vi>)  [unwired: 1 in]
  n26 = control-ref of="Tools"() -> (w75:refnum<vi>)
  n27 = control-ref of="Glyphs"() -> (w53:refnum<vi>)
  n28 = control-ref of="Templates"() -> (w54:refnum<vi>)
  n29 = control-ref of="Glyphs"() -> (w55:refnum<vi>)
  n30 = control-ref of="Font"() -> (w32:refnum<vi>)
  n31 = disable-structure shown="Disabled" {
    disable-tunnel: [w105 _] -> w23
    frame Disabled {
      # "Run this code to empty the combo box\nbefore saving this VI, if desired."
      n32 = control-ref of="Font"() -> (w108:refnum<vi>)
      n33 = property class="CmbBox (strict)"(reference=w108, "Strings[]"=string[] [] ("Strings []")) -> (error out=w106:errorcluster)  [unwired: 1 in, 1 out]
      n34 = invoke class="VI" method="Abort VI"(error in=w106) -> (error out=w105:errorcluster)  [unwired: 2 in, 2 out]
    }
    frame Enabled {
    }
  }
  n35 = control-ref of="Line Color"() -> (w73:refnum<vi>)
  n36 = control-ref of="Fill Color"() -> (w74:refnum<vi>)
  n37 = control-ref of="refreshGlyphs"() -> (w19:refnum<vi>)
  n38 = control-ref of="refreshTemplates"() -> (w20:refnum<vi>)
  n39 = control-ref of="Move Up"() -> (w50:refnum<vi>)
  n40 = control-ref of="Move Down"() -> (w51:refnum<vi>)
  n41 = control-ref of="Add Layer"() -> (w38:refnum<vi>)
  n42 = control-ref of="Remove Layer"() -> (w39:refnum<vi>)
  n43 = control-ref of="Body Text Spec"() -> (w47:refnum<vi>)
  n44 = control-ref of="Icon Text"() -> (w57:refnum<vi>)
  n45 = control-ref of="Icon Template"() -> (w58:refnum<vi>)
  n46 = control-ref of="Color icon in"() -> (w35:refnum<vi>)
  n47 = control-ref of="Color icon in"() -> (w62:refnum<vi>)
  n48 = control-ref of="User Layers"() -> (w64:refnum<vi>)
  n49 = control-ref of="Body Text"() -> (w66:refnum<vi>)
  n50 = control-ref of="DNL_Framework Templates"() -> (w69:refnum<vi>)
  n51 = control-ref of="Clipboard"() -> (w60:refnum<vi>)
  n52 = control-ref of="Icon"() -> (w76:refnum<vi>)
  n53 = control-ref of="Preview"() -> (w77:refnum<vi>)
  n54 = control-ref of="Preview2"() -> (w46:refnum<vi>)
  n55 = control-ref of="Terminals"() -> (w65:refnum<vi>)
  n56 = control-ref of="IE VI Ref"() -> (w52:refnum<vi>)
  n57 = control-ref of="LayerName"() -> (w26:refnum<vi>)
  n58 = control-ref of="LayerName"() -> (w27:refnum<vi>)
  n59 = control-ref of="LayerName"() -> (w28:refnum<vi>)
  n60 = control-ref of="LayerName"() -> (w29:refnum<vi>)
  n61 = control-ref of="Line 3 text"() -> (w43:refnum<vi>)
  n62 = control-ref of="Line 4 text"() -> (w44:refnum<vi>)
  n63 = control-ref of="glyph path str"() -> (w48:refnum<vi>)
  n64 = control-ref of="templates path str"() -> (w49:refnum<vi>)
  n65 = control-ref of="Filter templates by keyword"() -> (w70:refnum<vi>)
  n66 = control-ref of="TextMarker"() -> (w71:refnum<vi>)
  n67 = control-ref of="Filter glyphs by keyword"() -> (w72:refnum<vi>)
  n68 = control-ref of="Line 1 text"() -> (w41:refnum<vi>)
  n69 = control-ref of="Line 2 text"() -> (w42:refnum<vi>)
  n70 = control-ref of="Glyphs []"() -> (w36:refnum<vi>)
  n71 = Current VI's Menubar() -> (w63:refnum<k9>)
  n72 = Build Array(w41, w42, w43, w44) -> (w40:refnum<vi>[])
  n73 = Build Array(w26, w27, w28, w29) -> (w24:refnum<vi>[])
  n74 = Bundle(cluster=T23 {"Add Layer"=refnum, "Remove Layer"=refnum, "Line Text"=[], "Body Text Spec"=refnum, "DNL_Font"=refnum, "glyph path str"=refnum, "templates path str"=refnum, "Arrow Up"=refnum, "Arrow Down"=refnum, "IE VI Ref"=refnum, "Glyphs tree"=refnum, "Templates tree"=refnum, "Layer Icon Text"=refnum, "Layer Template"=refnum, "Clipboard"=refnum, "BW icon in"=refnum, "Color icon in"=refnum, "Layer Clust"=refnum, "Body Text"=refnum, "DNL_Framework Templates"=refnum, "Search Templates"=refnum, "TextMarker"=refnum, "Tab Control"=refnum, "Search Glyphs"=refnum, "Line Color"=refnum, "DNL_Glyphs []"=refnum, "Fill Color"=refnum, "Tools"=refnum, "Glyphs tree"=refnum, "Icon"=refnum, "Preview"=refnum, "Ants"=refnum, "Terminals"=refnum, "menu reference"=refnum, "LayerNames"=[], "GlyphLoadAnimation"=refnum, "TemplateLoadAnimation"=refnum, "refreshGlyphs"=refnum, "refreshTemplates"=refnum} ("references"), "Add Layer"=w38, "Remove Layer"=w39, "Line Text"=w40, "Body Text Spec"=w47, "DNL_Font"=w32, "glyph path str"=w48, "templates path str"=w49, "Arrow Up"=w50, "Arrow Down"=w51, "IE VI Ref"=w52, "Glyphs tree"=w53, "Templates tree"=w54, "Layer Icon Text"=w57, "Layer Template"=w58, "Clipboard"=w60, "BW icon in"=w35, "Color icon in"=w62, "Layer Clust"=w64, "Body Text"=w66, "DNL_Framework Templates"=w69, "Search Templates"=w70, "TextMarker"=w71, "Tab Control"=w18, "Search Glyphs"=w72, "Line Color"=w73, "DNL_Glyphs []"=w36, "Fill Color"=w74, "Tools"=w75, "Glyphs tree"=w55, "Icon"=w76, "Preview"=w77, "Ants"=w46, "Terminals"=w65, "menu reference"=w63, "LayerNames"=w24, "GlyphLoadAnimation"=w10, "TemplateLoadAnimation"=w11, "refreshGlyphs"=w19, "refreshTemplates"=w20) -> (w25:T23)
  n75 = property on="OK" class="Bool"(error in=w23, "KeyNav"=T24 {"Control"=FALSE, "Shift"=FALSE, "Key"="<Return>"} ("Key Navigation")) -> (error out=w33:errorcluster)  [unwired: 1 in, 1 out]
  n76 = call <resource>:"Initialization_UserEvents.vi"("error in (no error)"=w33, "References"=w25) -> ("error out"=w59:errorcluster, "Events"=w68:refnum<event-registration>, "User events"=w22:T27)  [unwired: 7 out]
  n77 = call <resource>:"Classes Initialization.vi"("LabVIEW Icon in"="LabVIEW Icon in", "error in (no error)"=w59, "User events"=w22, "Ref Cluster"=w25) -> ("error out"=w7:errorcluster, "Data out"=w45:T28)  [unwired: 1 in, 5 out]
  n78 = flat-sequence {
    tunnel: w7 -> [w109]
    tunnel: w2 -> [_]
    frame #0 {
      n79 = invoke class="VI" method="FP.Open"(error in=w109, "Activate"=TRUE ("Activate?")) -> ()  [unwired: 3 in, 5 out]
    }
  }
  n80 = Bundle("Events"=w68) -> (w67:cluster{"Events":refnum<event-registration>})  [unwired: 1 in]
  n81 = case shown="No Error" w7 {
    selector: w7 -> [w125 w844]
    tunnel: w67 -> [w143 _]
    tunnel: [w141 w845] -> w61
    tunnel: [w138 _] -> w56
    tunnel: w22 -> [w131 _]
    tunnel: w45 -> [w130 _]
    tunnel: w25 -> [w128 _]
    tunnel: [w127 _] -> w37
    tunnel: "LabVIEW Icon in" -> [w120 w843]
    tunnel: [w123 w843] -> w30
    tunnel: w22 -> [w116 _]
    tunnel: w2 -> [w115 _]
    tunnel: w1 -> [w111 _]
    frame No Error {
      # "Make sure the Keep IE in Memory VI runs and completes before the main Icon Editor panel is closed."
      # "Running ants"
      n82 = Unbundle By Name(w130) -> ("Class.Ants"=w129:refnum<class "Ants.lvclass">)
      n83 = Obtain Queue(max queue size (-1, unlimited)=100, element data type=T31 {"Horizontal"=0, "Vertical"=0} ("Coords"), error in (no error)=w125) -> (queue out=w132:refnum<queue>, error out=w133:errorcluster)  [unwired: 1 in, 2 out]
      n84 = while {
        shift-right: [w153] -> w122
        shift-left: w125 -> [w161]
        tunnel: [w157] -> w144
        tunnel: w143 -> [w156]
        tunnel: [w155] -> w140
        tunnel: w132 -> [w150]
        tunnel: w131 -> [w149]
        shift-right: [w146] -> w124
        shift-left: w130 -> [w148]
        border: T31 {"Horizontal"=-1, "Vertical"=-1} ("Corrected Out") -> [_]
        tunnel: w116 -> [w145]
        stop <- w158 stop-if-true
        n85 = event shown="[5] \"Execute custom override\", \"Class path\", \"Use PPL\": Value Change" {
          selector: w156 -> [_ _ _ _ _ _ _ _ _ _ _ _ _ _ _ _ _ _ _ _ _ _ _ _ _ _ _ _ _ _ _ _ _ _ _ _ _ _ _ _ _ _ _ _ _ _ _ _ _ _ _ _]
          dyn-events: [_ _ _ _ _ _ _ _ _ _ _ _ _ _ _ _ _ _ _ _ _ _ _ _ _ _ _ _ _ _ _ _ _ _ _ _ _ _ _ _ _ _ _ _ _ _ _ _ _ _ _ _] -> w157
          timeout: _ -> [_ _ _ _ _ _ _ _ _ _ _ _ _ _ _ _ _ _ _ _ _ _ _ _ _ _ _ _ _ _ _ _ _ _ _ _ _ _ _ _ _ _ _ _ _ _ _ _ _ _ _ _]
          tunnel: [w177 errorcluster {"status"=TRUE, "code"=43, "source"=""} ("error out") w193 w216 w234 w245 w250 w270 w292 w308 w324 w328 w342 w360 w367 w377 w385 w395 w405 w421 w429 w448 w462 w470 w488 w503 w518 w531 w549 w569 w576 w592 w602 w613 w616 w625 w639 w648 w660 w677 w687 w698 w701 w710 w723 errorcluster {"status"=TRUE, "code"=43, "source"=""} ("error out") w747 w777 w793 w798 w805 w812] -> w154
          tunnel: w161 -> [w179 _ w195 w218 w236 w244 w255 w282 w286 w309 w325 w331 w343 w361 w366 w376 w387 w398 w413 w425 w438 w455 w463 w475 w493 w506 w524 w545 w557 w569 w575 w593 w605 w613 w617 w634 w642 w651 w662 w681 w688 w698 w702 w714 w726 _ w753 w781 w794 w799 w806 w813]
          tunnel: [TRUE w186 _ _ _ _ _ _ _ _ _ _ _ _ _ _ _ _ _ _ _ _ _ _ _ _ _ _ _ _ _ _ _ _ _ _ _ _ _ _ _ _ _ _ _ w741 _ _ _ _ _ _] -> w159
          tunnel: "Tools" -> [_ _ w189 _ _ _ _ _ _ _ w323 _ _ _ _ _ _ _ _ _ _ _ _ _ _ _ _ _ _ _ _ _ _ _ _ _ _ _ _ _ _ _ _ _ _ _ _ _ _ _ _ _]
          tunnel: [TRUE w186 TRUE TRUE _ _ TRUE TRUE TRUE TRUE TRUE TRUE TRUE TRUE TRUE _ TRUE _ _ TRUE _ _ TRUE TRUE TRUE _ TRUE _ _ _ _ _ TRUE _ _ TRUE _ _ TRUE TRUE _ _ _ _ TRUE w741 TRUE ("Yes") TRUE _ _ _ _] -> w151
          tunnel: w150 -> [_ _ _ _ _ _ _ _ _ w306 _ _ _ _ _ _ _ _ _ _ _ _ _ _ _ _ _ _ _ _ _ _ _ _ _ _ _ _ _ _ _ _ _ _ _ _ _ _ _ _ _ _]
          tunnel: w149 -> [_ _ w192 _ _ _ _ _ _ _ _ _ _ _ _ _ _ _ _ _ _ _ _ _ _ _ _ _ _ _ _ _ _ _ _ _ _ _ _ _ _ _ _ _ _ _ _ _ _ _ _ _]
          tunnel: w148 -> [w176 w185 w191 w214 w233 w247 w254 w278 w288 w305 w321 w327 w338 w357 w365 w375 w380 w391 w403 w417 w434 w453 w460 w466 w484 w501 w516 w536 w554 w568 w573 w582 w600 w611 w614 w621 w638 w647 w658 w680 w685 w695 w704 w716 w733 w743 w752 w774 w796 w800 w803 w810]
          tunnel: [w172 w185 w190 w212 w232 w247 w259 w271 w291 w304 w319 w326 w335 w356 w363 w373 w381 w390 w407 w416 w430 w447 w459 w464 w482 w500 w515 w529 w550 w568 w571 w580 w599 w611 w615 w626 w637 w646 w652 w675 w684 w697 w704 w708 w719 w743 w745 w771 w795 w800 w803 w810] -> w147
          tunnel: [_ _ _ _ _ _ _ _ _ _ _ _ w332 _ _ _ _ _ _ _ _ _ _ _ _ _ _ _ _ _ _ _ _ _ _ _ _ _ _ _ _ _ _ _ _ _ _ _ _ _ _ _] -> _
          tunnel: w145 -> [_ _ _ _ _ _ _ _ _ _ _ _ _ _ _ _ _ _ _ _ _ _ _ _ _ _ _ _ _ _ _ _ _ _ _ _ _ _ _ _ _ _ _ _ _ _ _ _ _ _ w804 w811]
          event "OK": Value Change {
            n86 = event-data() -> ()  [unwired: 2 out]
            n87 = call <resource>:"Finalize Text.vi"("error in (no error)"=w179, "Data in"=w176) -> ("error out"=w180:errorcluster, "Data out"=w175:T28)  [unwired: 8 out]
            n88 = call <resource>:"Finalize Movement.vi"("error in (no error)"=w180, "Data in"=w175) -> ("error out"=w181:errorcluster, "Data out"=w174:T28)  [unwired: 1 in, 7 out]
            n89 = call <resource>:"DeselectLayer.vi"("error in (no error)"=w181, "Data in"=w174) -> ("error out"=w178:errorcluster, "Data out"=w173:T28)  [unwired: 8 out]
            n90 = call <resource>:"Reset layer template selection.vi"("error in (no error)"=w178, "Data in"=w173) -> ("error out"=w177:errorcluster, "Data out"=w172:T28)  [unwired: 1 in, 7 out]
          }
          event "Cancel": Value Change {
            w186 = FALSE ("Yes")
            n91 = event-data() -> ()  [unwired: 2 out]
          }
          event Menu Selection (User); Menu Selection (App) {
            n92 = event-data() -> ("Type"=w196:T34, "ItemTag"=w197:string)  [unwired: 1 out]
            n93 = case shown="\"Text\"" w189 {
              tunnel: w195 -> [w198 w203]
              tunnel: w191 -> [w199 w202]
              tunnel: [w198 w201] -> w187
              tunnel: [w199 w200] -> w188
              frame Default {
              }
              frame "Text" {
                n94 = call <resource>:"Finalize Text.vi"("error in (no error)"=w203, "Data in"=w202) -> ("error out"=w201:errorcluster, "Data out"=w200:T28)  [unwired: 8 out]
              }
            }
            n95 = case shown="\"Menu Selection (User)\"" w196 {
              tunnel: w197 -> [_ w211]
              tunnel: [w205 w210] -> w193
              tunnel: w187 -> [w205 w209]
              tunnel: w192 -> [_ w208]
              tunnel: w188 -> [w204 w207]
              tunnel: [w204 w206] -> w190
              frame Default {
              }
              frame "Menu Selection (User)" {
                n96 = call <resource>:"MenuSelection(User).vi"("User events"=w208, "error in"=w209, "ItemTag"=w211, "Data in"=w207) -> ("error out"=w210:errorcluster, "Data out"=w206:T28)  [unwired: 1 in, 5 out]
              }
            }
          }
          event Mouse Down {
            n97 = event-data() -> ("CtlRef"=w217:refnum<vi>, "Button"=w213:u16)  [unwired: 1 out]
            n98 = case shown="1, 2" w213 {
              tunnel: w218 -> [w220 w227]
              tunnel: w217 -> [_ w231]
              tunnel: [w220 w225] -> w216
              tunnel: w214 -> [w219 w222]
              tunnel: [w219 w221] -> w212
              frame 0, Default {
              }
              frame 1, 2 {
                n99 = control-ref of="This VI"() -> (w230:refnum<vi>)
                n100 = call <resource>:"Defer_FP_Updates.vi"("Defer Panel Updates"=TRUE, "error in (no error)"=w227, "lv_icon.vi in"=w230) -> ("error out"=w228:errorcluster, "lv icon.vi out"=w223:refnum<vi>)  [unwired: 7 out]
                n101 = call <resource>:"Template_MouseDown.vi"("Add to Undo?"=TRUE, "error in"=w228, "CtlRef"=w231, "Data in"=w222) -> ("error out"=w226:errorcluster, "Data out"=w221:T28)  [unwired: 1 in, 5 out]
                n102 = call <resource>:"Defer_FP_Updates.vi"("error in (no error)"=w226, "lv_icon.vi in"=w223) -> ("error out"=w225:errorcluster)  [unwired: 1 in, 8 out]
              }
            }
          }
          event Value Change {
            n103 = event-data() -> ("NewVal"=w235:T21)  [unwired: 1 out]
            n104 = call <resource>:"Value Change_Tools.vi"("error in"=w236, "NewVal"=w235, "Data in"=w233) -> ("error out"=w234:errorcluster, "Data out"=w232:T28)  [unwired: 7 out]
          }
          event "Execute custom override", "Class path", "Use PPL": Value Change {
            n105 = event-data() -> ()  [unwired: 7 out]
            n106 = Select(t=path "C:/git/labview-icon-editor/resource/plugins/PluginHarness.lvlibp/PluginHarness.lvclass" ("f"), s="Use PPL", f=path "C:/git/labview-icon-editor/Sandbox/Plugin harness/PluginHarness.lvclass" ("Class path")) -> (s? t:f=w242:path)
            "Class path" <- w242
            n107 = call <vilib>:"Execute action.vi"("error in (no error)"=w244, "vi path"=path "C:/git/labview-icon-editor/resource/plugins/IconEditorInterface.lvlibp/Harness - Action.vi", "Action"="Action", "Class path"=w242) -> ("error out"=w241:errorcluster)  [unwired: 7 in]
            n108 = call <vilib>:"Simple Error Handler.vi"("error in (no error)"=w241) -> ("error out"=w240:errorcluster)  [unwired: 4 in, 4 out]
            n109 = flat-sequence {
              tunnel: [w248] -> w245
              tunnel: w244 -> [w248]
              tunnel: w240 -> [_]
              frame #0 {
              }
            }
          }
          event Mouse Down {
            n110 = event-data() -> ("Mods.Double Click"=w249:bool)  [unwired: 1 out]
            n111 = call <resource>:"Finalize Text.vi"("error in (no error)"=w255, "Data in"=w254) -> ("error out"=w257:errorcluster, "Data out"=w256:T28)  [unwired: 8 out]
            n112 = call <resource>:"Finalize Movement.vi"("error in (no error)"=w257, "Data in"=w256) -> ("error out"=w253:errorcluster, "Data out"=w252:T28)  [unwired: 1 in, 7 out]
            n113 = call <resource>:"Mouse Down.vi"("error in"=w253, "Double Click"=w249, "Data in"=w252) -> ("error out"=w250:errorcluster, "Data out"=w251:T28)  [unwired: 7 out]
            n114 = Bundle By Name(cluster=w251, "Support.Tool (old value)"=u32 111) -> (w259:T28)
          }
          event Value Change {
            # "Body Text Value Change event is fired programmatically during initialization so first call of this event is guaranteed to be a case we do not want to update the undo/redo information."
            n115 = event-data() -> ("OldVal"=w269:T8, "NewVal"=w268:T8, "OldVal.Body Text Spec.Alignment"=w273:T10)  [unwired: 1 out]
            n116 = Unbundle By Name(w269) -> ("Body Text Spec.Font"=w267:T9)
            n117 = Unbundle By Name(w268) -> ("Body Text Spec.Font"=w266:T9)
            n118 = local read "Tab Control"() -> (w264:T5)
            n119 = Unbundle By Name(w268) -> ("Body Text Spec.Alignment"=w274:T10)
            n120 = First Call?() -> (First Call?: T/F=w281:bool)
            n121 = Equal?(x=w264, y=T5."Icon Text") -> (x = y?=w262:bool)
            n122 = Not(x=w281) -> (.not. x?=w280:bool)
            n123 = Not Equal?(x=w267, y=w266) -> (x != y?=w265:bool)
            n124 = call <resource>:"Value Change_Body Text.vi"("Layer Icon"="Icon Text", "Add to Undo?"=w280, "error in"=w282, "NewVal"=w268, "Data in"=w278) -> ("error out"=w276:errorcluster, "Data out"=w275:T28)  [unwired: 5 out]
            n125 = And(x=w262, y=w265) -> (x .and. y?=w261:bool)
            n126 = Not Equal?(x=w274, y=w273) -> (x != y?=w272:bool)
            n127 = case shown="True" w261 {
              frame False {
              }
              frame True {
                n128 = property on="Line 1 text" class="Str"("Key Focus"=TRUE) -> ()  [unwired: 2 in, 2 out]
              }
            }
            n129 = call <resource>:"Alignment Value Change.vi"("Set Focus?"=w272, "error in"=w276, "NewVal"=w274, "Data in"=w275) -> ("error out"=w270:errorcluster, "Data out"=w271:T28)  [unwired: 6 out]
          }
          event Value Change {
            n130 = event-data() -> ()  [unwired: 2 out]
            n131 = call <resource>:"Finalize Text.vi"("error in (no error)"=w286, "Data in"=w288) -> ("error out"=w290:errorcluster, "Data out"=w289:T28)  [unwired: 8 out]
            n132 = local read "Line Color"() -> (w285:T20)
            n133 = local read "Fill Color"() -> (w295:T20)
            n134 = call <resource>:"Finalize Movement.vi"("error in (no error)"=w290, "Data in"=w289) -> ("error out"=w284:errorcluster, "Data out"=w287:T28)  [unwired: 1 in, 7 out]
            n135 = stacked-sequence {
              tunnel: w295 -> [w299]
              tunnel: [w298] -> w293
              tunnel: w285 -> [w297]
              tunnel: w284 -> [w296]
              frame #0 {
                n136 = local write "Fill Color"(w297) -> ()
                n137 = property on="Line Color" class="ColBox (strict)"(error in=w296, "Val(Sgnl)"=w299) -> (error out=w298:errorcluster)  [unwired: 1 in, 1 out]
              }
            }
            n138 = call <resource>:"Escape.vi"("error in"=w293, "Data in"=w287) -> ("error out"=w292:errorcluster, "Data out"=w291:T28)  [unwired: 1 in, 7 out]
          }
          event "Preview", "Terminals", "Preview2": Mouse Move {
            n139 = event-data() -> ("Coords"=w303:T31)  [unwired: 1 out]
            n140 = call <resource>:"CoordinatesCorrection.vi"("Coordinates In"=w303) -> ("Corrected Out"=w300:T31)  [unwired: 10 out]
            n141 = feedback-in #1(w300) -> ()
            n142 = feedback #1() -> (w302:T31)
            n143 = Not Equal?(x=w302, y=w300) -> (x != y?=w301:bool)
            n144 = case shown="True" w301 {
              tunnel: w309 -> [w311 w317]
              tunnel: [w311 w316] -> w308
              tunnel: w306 -> [_ w315]
              tunnel: w305 -> [w310 w314]
              tunnel: [w310 w313] -> w304
              tunnel: w300 -> [_ w312]
              frame False {
              }
              frame True {
                n145 = call <resource>:"MouseMove.vi"("Buffer"=w315, "error in"=w317, "Coords"=w312, "Data in"=w314) -> ("error out"=w316:errorcluster, "Data out"=w313:T28)  [unwired: 6 out]
              }
            }
          }
          event "Preview", "Terminals", "Preview2": Mouse Enter {
            n146 = event-data() -> ()  [unwired: 2 out]
            n147 = call <resource>:"SetCursor.vi"("error in (no error)"=w325, "Radio Buttons"=w323, "Data in"=w321) -> ("error out"=w324:errorcluster, "Data out"=w320:T28)  [unwired: 7 out]
            n148 = Bundle By Name(cluster=w320, "Support.Mouse inside icon?"=TRUE) -> (w319:T28)
          }
          event "Preview", "Terminals", "Preview2": Mouse Up {
            n149 = event-data() -> ("Coords"=w330:T31)  [unwired: 1 out]
            n150 = call <resource>:"PictureControl_MouseUp.vi"("error in"=w331, "Coords"=w330, "Data in"=w327) -> ("error out"=w328:errorcluster, "Data out"=w326:T28)  [unwired: 4 in, 3 out]
          }
          event Key Down?; event type 5.0.x8000000b {
            n151 = event-data() -> ("Type"=w337:T34, "Char"=w334:i16, "VKey"=w341:T35, "PlatMods"=w336:T36)  [unwired: 1 out]
            n152 = Equal?(x=i16 99, y=w334) -> (x = y?=w332:bool)
            n153 = call <resource>:"KeyDown.vi"("PlatMods"=w336, "Type"=w337, "error in (no error)"=w343, "VKey"=w341, "Char"=w334, "Data in"=w338) -> ("error out"=w342:errorcluster, "Discard?"=w340:bool, "Data out"=w335:T28)  [unwired: 3 out]
            n154 = event-data("Discard?"=w340) -> ()  [unwired: 1 in, 1 out]
          }
          event "Preview", "Terminals", "Preview2": Mouse Down {
            # "Left click"
            n155 = event-data() -> ("Button"=w346:u16, "Coords"=w359:T31)  [unwired: 1 out]
            n156 = Not Equal?(x=u16 1, y=w346) -> (x != y?=w344:bool)
            n157 = control-ref of="This VI"() -> (w355:refnum<vi>)
            n158 = call <resource>:"Defer_FP_Updates.vi"("Defer Panel Updates"=TRUE, "error in (no error)"=w361, "lv_icon.vi in"=w355) -> ("error out"=w351:errorcluster, "lv icon.vi out"=w353:refnum<vi>)  [unwired: 7 out]
            n159 = call <resource>:"Reset layer template selection.vi"("Force reset? (T)"=FALSE, "error in (no error)"=w351, "Data in"=w357) -> ("error out"=w350:errorcluster, "Data out"=w347:T28)  [unwired: 1 in, 6 out]
            n160 = call <resource>:"MouseDown.vi"("Flip colors?"=w344, "error in"=w350, "Coords"=w359, "Data in"=w347) -> ("error out"=w349:errorcluster, "Data out"=w356:T28)  [unwired: 1 in, 5 out]
            n161 = call <resource>:"Defer_FP_Updates.vi"("Defer Panel Updates"=FALSE, "error in (no error)"=w349, "lv_icon.vi in"=w353) -> ("error out"=w360:errorcluster)  [unwired: 8 out]
          }
          event Value Change {
            n162 = event-data() -> ()  [unwired: 2 out]
            n163 = call <vilib>:"Check Color.vi"("Color in"="Fill Color") -> ("Color out"=w368:T20)  [unwired: 26 out]
            n164 = call <vilib>:"Check Color.vi"("Color in"="Line Color") -> ("Color out"=w369:T20)  [unwired: 26 out]
            n165 = Bundle By Name(cluster=w365, "Support.Fill Color"=w368, "Support.Edge Color"=w369) -> (w364:T28)
            n166 = call <resource>:"Escape.vi"("Reset cursor (T)"=FALSE ("Reset cursor? (T)"), "error in"=w366, "Data in"=w364) -> ("error out"=w367:errorcluster, "Data out"=w363:T28)  [unwired: 1 in, 6 out]
          }
          event Key Up {
            n167 = event-data() -> ("PlatMods"=w374:T36)  [unwired: 1 out]
            n168 = call <resource>:"KeyUp.vi"("error in (no error)"=w376, "PlatMods"=w374, "Data in"=w375) -> ("error out"=w377:errorcluster, "Data out"=w373:T28)  [unwired: 7 out]
          }
          event Value Change {
            n169 = event-data() -> ()  [unwired: 2 out]
            n170 = call <resource>:"Finalize Text.vi"("error in (no error)"=w387, "Data in"=w380) -> ("error out"=w386:errorcluster, "Data out"=w382:T28)  [unwired: 8 out]
            n171 = call <resource>:"Finalize Movement.vi"("error in (no error)"=w386, "Data in"=w382) -> ("error out"=w383:errorcluster, "Data out"=w379:T28)  [unwired: 1 in, 7 out]
            n172 = call <resource>:"RotateFlip.vi"("error in"=w383, "Rotate"="Clockwise Rotate", "Data in"=w379) -> ("error out"=w384:errorcluster, "Data out"=w378:T28)  [unwired: 2 in, 5 out]
            n173 = call <resource>:"Escape.vi"("error in"=w384, "Data in"=w378) -> ("error out"=w385:errorcluster, "Data out"=w381:T28)  [unwired: 1 in, 7 out]
          }
          event Value Change {
            n174 = event-data() -> ("NewVal"=w400:variant)  [unwired: 1 out]
            n175 = control-ref of="This VI"() -> (w397:refnum<vi>)
            n176 = call <resource>:"Defer_FP_Updates.vi"("Defer Panel Updates"=TRUE, "error in (no error)"=w398, "lv_icon.vi in"=w397) -> ("error out"=w399:errorcluster, "lv icon.vi out"=w392:refnum<vi>)  [unwired: 7 out]
            n177 = call <resource>:"Mouse Down_Templates.vi"("Tag"="Templates", "error in"=w399, "NewVal"=w400, "Data in"=w391) -> ("error out"=w394:errorcluster, "Data out"=w390:T28)  [unwired: 1 in, 5 out]
            n178 = call <resource>:"Defer_FP_Updates.vi"("error in (no error)"=w394, "lv_icon.vi in"=w392) -> ("error out"=w395:errorcluster)  [unwired: 1 in, 8 out]
          }
          event User Event {
            # "This is an initialization event for the glyphs."
            n179 = event-data() -> ("Glyphs"=w415:string)  [unwired: 1 out]
            n180 = Unbundle By Name(w403) -> ("Ref.GlyphLoadAnimation"=w402:refnum<vi>, "Ref.refreshGlyphs"=w401:refnum<vi>)
            n181 = Unflatten From String(type="?", binary string=w415, error in (no error)=w413) -> (value=w410:T3[], error out=w412:errorcluster)  [unwired: 3 out]
            n182 = call <resource>:"Populate Graphics.vi"("error in"=w412, "Glyphs []"=w410, "Data in"=w403) -> ("error out"=w411:errorcluster, "Data out"=w407:T28)  [unwired: 7 out]
            n183 = call <resource>:"Write Glyphs to  File.vi"("File Name"="Glyphs.bin", "Path"=Pathes."Glyphs", "error in (no error)"=w411, "Graphics []"=w410) -> ("error out"=w406:errorcluster)  [unwired: 7 out]
            n184 = call <resource>:"ChangeRefreshGraphicsState.vi"("error in (no error)"=w406, "refreshing?"=FALSE, "button ref"=w401, "animatedDecoration ref"=w402) -> ("error out"=w405:errorcluster)  [unwired: 7 in]
          }
          event Mouse Down {
            n185 = event-data() -> ("PlatMods.Shift"=w418:bool, "CtlRef"=w428:refnum<vi>, "PlatMods.Ctrl"=w427:bool)  [unwired: 1 out]
            n186 = control-ref of="This VI"() -> (w424:refnum<vi>)
            n187 = call <resource>:"Defer_FP_Updates.vi"("Defer Panel Updates"=TRUE, "error in (no error)"=w425, "lv_icon.vi in"=w424) -> ("error out"=w423:errorcluster, "lv icon.vi out"=w420:refnum<vi>)  [unwired: 7 out]
            n188 = call <resource>:"Mouse Down_User Layers.vi"("Shift"=w418, "error in"=w423, "Ctrl"=w427, "CtlRef"=w428, "Data in"=w417) -> ("error out"=w422:errorcluster, "Data out"=w416:T28)  [unwired: 5 out]
            n189 = call <resource>:"Defer_FP_Updates.vi"("error in (no error)"=w422, "lv_icon.vi in"=w420) -> ("error out"=w421:errorcluster)  [unwired: 1 in, 8 out]
          }
          event "Filter glyphs by keyword": Mouse Down {
            # "If a mouse down event should\nselect the entered text, enable this case"
            n190 = event-data() -> ("CtlRef"=w437:refnum<vi>)  [unwired: 1 out]
            n191 = disable-structure shown="Enabled" {
              disable-tunnel: w438 -> [w441 w444]
              disable-tunnel: w437 -> [w440 _]
              disable-tunnel: [w439 w444] -> w436
              frame Disabled {
                n192 = property class="Str"(reference=w440, error in=w441, "Text.Selection Start"=u32 0 ("Text.Selection:Start"), "Text.Selection End"=-1 ("Text.Selection:End")) -> (error out=w439:errorcluster)  [unwired: 1 out]
              }
              frame Enabled {
              }
            }
            n193 = call <resource>:"Finalize Text.vi"("error in (no error)"=w436, "Data in"=w434) -> ("error out"=w435:errorcluster, "Data out"=w433:T28)  [unwired: 8 out]
            n194 = call <resource>:"DeselectLayer.vi"("error in (no error)"=w435, "Data in"=w433) -> ("error out"=w432:errorcluster, "Data out"=w431:T28)  [unwired: 8 out]
            n195 = call <resource>:"Escape.vi"("error in"=w432, "Data in"=w431) -> ("error out"=w429:errorcluster, "Data out"=w430:T28)  [unwired: 1 in, 7 out]
          }
          event "Filter glyphs by keyword": Value Change {
            n196 = event-data() -> ("NewVal"=w458:string)  [unwired: 1 out]
            n197 = Unbundle By Name(w453) -> ("Class.Glyph"=w454:refnum<class "Glyph.lvclass">, "Ref.DNL_Glyphs []"=w451:refnum<vi>, "Ref.Glyphs tree"=w450:refnum<vi>)
            n198 = First Call?() -> (First Call?: T/F=w456:bool)
            n199 = Not(x=w456) -> (.not. x?=w457:bool)
            n200 = call <resource>:"SearchGlyphs.vi"("Glyphs tree"=w450, "DNL_Glyphs []"=w451, "Reset position? (F)"=w457, "error in (no error)"=w455, "Keyword"=w458, "Glyph in"=w454) -> ("error out"=w449:errorcluster, "Glyph out"=w452:refnum<class "Glyph.lvclass">)  [unwired: 4 out]
            n201 = Bundle By Name(cluster=w453, "Class.Glyph"=w452) -> (w446:T28)
            n202 = call <resource>:"Add Data to History.vi"("Add to Undo?"=TRUE, "error in"=w449, "Data in"=w446) -> ("error out"=w448:errorcluster, "Data out"=w447:T28)  [unwired: 7 out]
          }
          event Mouse Down {
            n203 = event-data() -> ()  [unwired: 2 out]
            n204 = call <resource>:"MouseDown_Body Text.vi"("error in"=w463, "Data in"=w460) -> ("error out"=w462:errorcluster, "Data out"=w459:T28)  [unwired: 8 out]
          }
          event Value Change {
            n205 = event-data() -> ("OldVal.Opacity"=w469:u8, "NewVal.Opacity"=w468:u8, "NewVal"=w474:T15)  [unwired: 1 out]
            n206 = Not Equal?(x=w469, y=w468) -> (x != y?=w467:bool)
            n207 = call <resource>:"Value Change_Top or Bottom Layer.vi"("Type"=enum16{"Template Layer", "Text Layer"}."Text Layer", "error in (no error)"=w475, "Data"=w474, "Data in"=w466) -> ("error out"=w471:errorcluster, "Data out"=w465:T28)  [unwired: 6 out]
            n208 = case shown="True" w467 {
              tunnel: w471 -> [w477 w481]
              tunnel: [w477 w480] -> w470
              tunnel: w465 -> [w476 w479]
              tunnel: [w476 w478] -> w464
              frame False {
              }
              frame True {
                n209 = call <resource>:"Reset layer template selection.vi"("error in (no error)"=w481, "Data in"=w479) -> ("error out"=w480:errorcluster, "Data out"=w478:T28)  [unwired: 1 in, 7 out]
              }
            }
          }
          event Value Change {
            n210 = event-data() -> ("OldVal.Opacity"=w486:u8, "NewVal.Opacity"=w487:u8, "NewVal"=w491:T15)  [unwired: 1 out]
            n211 = Not Equal?(x=w486, y=w487) -> (x != y?=w485:bool)
            n212 = call <resource>:"Value Change_Top or Bottom Layer.vi"("Type"=enum16{"Template Layer", "Text Layer"}."Template Layer", "error in (no error)"=w493, "Data"=w491, "Data in"=w484) -> ("error out"=w489:errorcluster, "Data out"=w483:T28)  [unwired: 6 out]
            n213 = case shown="False" w485 {
              tunnel: w489 -> [w495 w499]
              tunnel: [w495 w498] -> w488
              tunnel: w483 -> [w494 w497]
              tunnel: [w494 w496] -> w482
              frame False {
              }
              frame True {
                n214 = call <resource>:"Reset layer template selection.vi"("error in (no error)"=w499, "Data in"=w497) -> ("error out"=w498:errorcluster, "Data out"=w496:T28)  [unwired: 1 in, 7 out]
              }
            }
          }
          event Value Change {
            n215 = event-data() -> ("NewVal"=w510:variant)  [unwired: 1 out]
            n216 = control-ref of="This VI"() -> (w507:refnum<vi>)
            n217 = call <resource>:"Defer_FP_Updates.vi"("Defer Panel Updates"=TRUE, "error in (no error)"=w506, "lv_icon.vi in"=w507) -> ("error out"=w505:errorcluster, "lv icon.vi out"=w502:refnum<vi>)  [unwired: 7 out]
            n218 = Variant To Data(error in=w505, type=0, Variant=w510) -> (data=w509:i32, error out=w511:errorcluster)
            n219 = call <resource>:"UpdateLayerView_ScrollbarChanged.vi"("error in"=w511, "Scrollbar Position"=w509, "Data in"=w501) -> ("error out"=w504:errorcluster, "Data out"=w500:T28)  [unwired: 7 out]
            n220 = call <resource>:"Defer_FP_Updates.vi"("error in (no error)"=w504, "lv_icon.vi in"=w502) -> ("error out"=w503:errorcluster)  [unwired: 1 in, 8 out]
          }
          event Value Change {
            # "We do not use the dynamic registerd event for Layer Clust.Value Change\nbecause it would be a huge effort to lock the front panel until this\nevent case has been completed."
            n221 = event-data() -> ("OldVal.Visibility?"=w514:bool, "CtlRef"=w528:refnum<vi>, "OldVal.LayerName"=w513:string)  [unwired: 1 out]
            n222 = control-ref of="This VI"() -> (w525:refnum<vi>)
            n223 = call <resource>:"Defer_FP_Updates.vi"("Defer Panel Updates"=TRUE, "error in (no error)"=w524, "lv_icon.vi in"=w525) -> ("error out"=w523:errorcluster, "lv icon.vi out"=w520:refnum<vi>)  [unwired: 7 out]
            n224 = call <resource>:"LayerCluster_ValueChange.vi"("Old Visibility?"=w514, "error in"=w523, "Old name"=w513, "CtlRef"=w528, "Data in"=w516) -> ("error out"=w522:errorcluster, "Data out"=w517:T28)  [unwired: 1 in, 4 out]
            n225 = call <resource>:"Defer_FP_Updates.vi"("Defer Panel Updates"=FALSE, "error in (no error)"=w522, "lv_icon.vi in"=w520) -> ("error out"=w519:errorcluster)  [unwired: 8 out]
            n226 = call <resource>:"Reset layer template selection.vi"("error in (no error)"=w519, "Data in"=w517) -> ("error out"=w518:errorcluster, "Data out"=w515:T28)  [unwired: 1 in, 7 out]
          }
          event "Filter templates by keyword": Value Change {
            n227 = event-data() -> ("NewVal"=w548:string)  [unwired: 1 out]
            n228 = Unbundle By Name(w536) -> ("Ref.Templates tree"=w534:refnum<vi>, "Class.Templates"=w537:refnum<class "FakedArray.lvclass">)
            n229 = control-ref of="This VI"() -> (w547:refnum<vi>)
            n230 = call <resource>:"Defer_FP_Updates.vi"("Defer Panel Updates"=TRUE, "error in (no error)"=w545, "lv_icon.vi in"=w547) -> ("error out"=w539:errorcluster, "lv icon.vi out"=w544:refnum<vi>)  [unwired: 7 out]
            n231 = call-dynamic "SET_ScrollbarPosition.vi"("error in (no error)"=w539, "FakedArray.lvclass in"=w537) -> ("error out"=w540:errorcluster, "FakedArray.lvclass out"=w541:refnum<class "FakedArray.lvclass">)  [unwired: 1 in, 7 out]
            n232 = call <resource>:"ResetColor.vi"("error in (no error)"=w540, "FakedArray in"=w541) -> ("error out"=w542:errorcluster, "FakedArray out"=w543:refnum<class "FakedArray.lvclass">)  [unwired: 8 out]
            n233 = call-dynamic "UpdateVisibleData.vi"("Templates tree"=w534, "error in (no error)"=w542, "Keyword"=w548, "FakedArray in"=w543) -> ("error out"=w538:errorcluster, "FakedArray out"=w535:refnum<class "FakedArray.lvclass">)  [unwired: 1 in, 5 out]
            n234 = Bundle By Name(cluster=w536, "Class.Templates"=w535) -> (w530:T28)
            n235 = call <resource>:"Defer_FP_Updates.vi"("error in (no error)"=w538, "lv_icon.vi in"=w544) -> ("error out"=w532:errorcluster)  [unwired: 1 in, 8 out]
            n236 = call <resource>:"Add Data to History.vi"("Add to Undo?"=TRUE, "error in"=w532, "Data in"=w530) -> ("error out"=w531:errorcluster, "Data out"=w529:T28)  [unwired: 7 out]
          }
          event "Filter templates by keyword": Mouse Down {
            # "If a mouse down event should\nselect the entered text, enable this case"
            n237 = event-data() -> ("CtlRef"=w558:refnum<vi>)  [unwired: 1 out]
            n238 = disable-structure shown="Enabled" {
              disable-tunnel: w558 -> [w563 _]
              disable-tunnel: w557 -> [w561 w564]
              disable-tunnel: [w559 w564] -> w556
              frame Disabled {
                n239 = property class="Str"(reference=w563, error in=w561, "Text.Selection Start"=u32 0 ("Text.Selection:Start"), "Text.Selection End"=-1 ("Text.Selection:End")) -> (error out=w559:errorcluster)  [unwired: 1 out]
              }
              frame Enabled {
              }
            }
            n240 = call <resource>:"Finalize Text.vi"("error in (no error)"=w556, "Data in"=w554) -> ("error out"=w555:errorcluster, "Data out"=w553:T28)  [unwired: 8 out]
            n241 = call <resource>:"DeselectLayer.vi"("error in (no error)"=w555, "Data in"=w553) -> ("error out"=w552:errorcluster, "Data out"=w551:T28)  [unwired: 8 out]
            n242 = call <resource>:"Escape.vi"("error in"=w552, "Data in"=w551) -> ("error out"=w549:errorcluster, "Data out"=w550:T28)  [unwired: 1 in, 7 out]
          }
          event "Help": Value Change {
            n243 = event-data() -> ()  [unwired: 2 out]
            n244 = control-ref of="This VI"() -> (w567:refnum<vi>)
            n245 = property class="VI"(reference=w567) -> (error out=w565:errorcluster, "Help.URL"=w566:string)  [unwired: 1 in, 1 out]
            n246 = call <resource>:"IE_Open Help Link.vi"("error in (no error)"=w565, "Help.URL"=w566) -> ()  [unwired: 9 in, 1 out]
          }
          event "Glyphs": Value Change {
            n247 = event-data() -> ("NewVal"=w577:string)  [unwired: 1 out]
            n248 = Unbundle By Name(w573) -> ("Class.Glyph"=w574:refnum<class "Glyph.lvclass">, "Ref.DNL_Glyphs []"=w570:refnum<vi>)
            n249 = call <resource>:"FilterGlyphs.vi"("error in (no error)"=w575, "DNL_Glyphs []"=w570, "Tag"=w577, "Glyph in"=w574) -> ("error out"=w576:errorcluster, "Glyph out"=w572:refnum<class "Glyph.lvclass">)  [unwired: 6 out]
            n250 = Bundle By Name(cluster=w573, "Class.Glyph"=w572) -> (w571:T28)
          }
          event "Templates": Value Change {
            n251 = event-data() -> ("CtlRef"=w579:refnum<vi>, "NewVal"=w591:string)  [unwired: 1 out]
            n252 = control-ref of="This VI"() -> (w595:refnum<vi>)
            n253 = Unbundle By Name(w582) -> ("Class.Templates"=w583:refnum<class "FakedArray.lvclass">)
            n254 = call <resource>:"Defer_FP_Updates.vi"("Defer Panel Updates"=TRUE, "error in (no error)"=w593, "lv_icon.vi in"=w595) -> ("error out"=w585:errorcluster, "lv icon.vi out"=w590:refnum<vi>)  [unwired: 7 out]
            n255 = call-dynamic "SET_ScrollbarPosition.vi"("error in (no error)"=w585, "FakedArray.lvclass in"=w583) -> ("error out"=w587:errorcluster, "FakedArray.lvclass out"=w586:refnum<class "FakedArray.lvclass">)  [unwired: 1 in, 7 out]
            n256 = local write "Filter templates by keyword"("") -> ()
            n257 = call <resource>:"ResetColor.vi"("error in (no error)"=w587, "FakedArray in"=w586) -> ("error out"=w588:errorcluster, "FakedArray out"=w589:refnum<class "FakedArray.lvclass">)  [unwired: 8 out]
            n258 = call-dynamic "UpdateVisibleData.vi"("Templates tree"=w579, "error in (no error)"=w588, "Tag"=w591, "FakedArray in"=w589) -> ("error out"=w584:errorcluster, "FakedArray out"=w581:refnum<class "FakedArray.lvclass">)  [unwired: 1 in, 5 out]
            n259 = Bundle By Name(cluster=w582, "Class.Templates"=w581) -> (w580:T28)
            n260 = call <resource>:"Defer_FP_Updates.vi"("error in (no error)"=w584, "lv_icon.vi in"=w590) -> ("error out"=w592:errorcluster)  [unwired: 1 in, 8 out]
          }
          event Value Change {
            n261 = event-data() -> ()  [unwired: 2 out]
            n262 = control-ref of="This VI"() -> (w606:refnum<vi>)
            n263 = call <resource>:"Defer_FP_Updates.vi"("Defer Panel Updates"=TRUE, "error in (no error)"=w605, "lv_icon.vi in"=w606) -> ("error out"=w604:errorcluster, "lv icon.vi out"=w603:refnum<vi>)  [unwired: 7 out]
            n264 = call <resource>:"MoveLayers.vi"("error in"=w604, "Arrow Up"="Move Up", "Data in"=w600) -> ("error out"=w596:errorcluster, "Data out"=w599:T28)  [unwired: 7 out]
            n265 = stacked-sequence {
              tunnel: [w609] -> w597
              tunnel: w596 -> [w609]
              frame #0 {
                w610 = FALSE ("Arrow Down")
                n266 = local write "Move Down"(w610) -> ()
                n267 = local write "Move Up"(w610) -> ()
              }
            }
            n268 = call <resource>:"Defer_FP_Updates.vi"("Defer Panel Updates"=FALSE, "error in (no error)"=w597, "lv_icon.vi in"=w603) -> ("error out"=w602:errorcluster)  [unwired: 8 out]
          }
          event Shortcut Menu Activation? {
            n269 = event-data() -> ()  [unwired: 2 out]
            n270 = event-data("Discard?"=TRUE) -> ()  [unwired: 1 in, 1 out]
          }
          event Mouse Leave; Mouse Up {
            n271 = event-data() -> ()  [unwired: 2 out]
            n272 = call <resource>:"Add Data to History.vi"("Add to Undo?"=TRUE, "error in"=w617, "Data in"=w614) -> ("error out"=w616:errorcluster, "Data out"=w615:T28)  [unwired: 7 out]
          }
          event User Event {
            # "This is an initialization event for the templates"
            n273 = event-data() -> ("Templates"=w636:string)  [unwired: 1 out]
            n274 = Unbundle By Name(w621) -> ("Ref.TemplateLoadAnimation"=w620:refnum<vi>, "Ref.refreshTemplates"=w619:refnum<vi>)
            n275 = control-ref of="This VI"() -> (w631:refnum<vi>)
            n276 = call <resource>:"Defer_FP_Updates.vi"("Defer Panel Updates"=TRUE, "error in (no error)"=w634, "lv_icon.vi in"=w631) -> ("error out"=w629:errorcluster, "lv icon.vi out"=w628:refnum<vi>)  [unwired: 7 out]
            n277 = Unflatten From String(type="?", binary string=w636, error in (no error)=w629) -> (value=w627:cluster{T1[], i32, bool}, error out=w632:errorcluster)  [unwired: 3 out]
            n278 = call <resource>:"Process Template Graphics.vi"("error in (no error)"=w632, "Data"=w627, "Data in"=w621) -> ("error out"=w624:errorcluster, "Data out"=w626:T28)  [unwired: 7 out]
            n279 = call <resource>:"ChangeRefreshGraphicsState.vi"("error in (no error)"=w624, "refreshing?"=FALSE, "button ref"=w619, "animatedDecoration ref"=w620) -> ("error out"=w623:errorcluster)  [unwired: 7 in]
            n280 = call <resource>:"Defer_FP_Updates.vi"("error in (no error)"=w623, "lv_icon.vi in"=w628) -> ("error out"=w625:errorcluster)  [unwired: 1 in, 8 out]
          }
          event "Templates": Mouse Down {
            n281 = event-data() -> ("CtlRef"=w641:refnum<vi>, "Coords"=w643:T31)  [unwired: 1 out]
            n282 = call <resource>:"Mouse Down_Tree.vi"("Tree"=w641, "error in (no error)"=w642, "Coords"=w643) -> ("error out"=w640:errorcluster)  [unwired: 8 out]
            n283 = call <resource>:"Escape.vi"("error in"=w640, "Data in"=w638) -> ("error out"=w639:errorcluster, "Data out"=w637:T28)  [unwired: 1 in, 7 out]
          }
          event "Glyphs": Mouse Down {
            n284 = event-data() -> ("CtlRef"=w645:refnum<vi>, "Coords"=w650:T31)  [unwired: 1 out]
            n285 = local write "Filter glyphs by keyword"("") -> ()
            n286 = call <resource>:"Mouse Down_Tree.vi"("Tree"=w645, "error in (no error)"=w651, "Coords"=w650) -> ("error out"=w649:errorcluster)  [unwired: 8 out]
            n287 = call <resource>:"Escape.vi"("error in"=w649, "Data in"=w647) -> ("error out"=w648:errorcluster, "Data out"=w646:T28)  [unwired: 1 in, 7 out]
          }
          event "Tab Control": Value Change {
            n288 = event-data() -> ("NewVal"=w663:T5)  [unwired: 1 out]
            n289 = case shown="\"Templates\"" w663 {
              tunnel: w662 -> [w667 w670 w672 w674]
              tunnel: [w666 w669 w673 w674] -> w661
              frame "Templates" {
                n290 = property on="Filter templates by keyword" class="Str"(error in=w667, "Key Focus"=TRUE) -> (error out=w666:errorcluster)  [unwired: 1 in, 1 out]
              }
              frame "Glyphs" {
                n291 = property on="Filter glyphs by keyword" class="Str"(error in=w670, "Key Focus"=TRUE) -> (error out=w669:errorcluster)  [unwired: 1 in, 1 out]
              }
              frame "Icon Text" {
                n292 = property on="Line 1 text" class="Str"(error in=w672, "Key Focus"=TRUE) -> (error out=w673:errorcluster)  [unwired: 1 in, 1 out]
              }
              frame "Layers", Default {
              }
            }
            n293 = call <resource>:"Finalize Text.vi"("error in (no error)"=w661, "Data in"=w658) -> ("error out"=w664:errorcluster, "Data out"=w657:T28)  [unwired: 8 out]
            n294 = call <resource>:"Finalize Movement.vi"("error in (no error)"=w664, "Data in"=w657) -> ("error out"=w656:errorcluster, "Data out"=w654:T28)  [unwired: 1 in, 7 out]
            n295 = call <resource>:"Escape.vi"("error in"=w656, "Data in"=w654) -> ("error out"=w655:errorcluster, "Data out"=w653:T28)  [unwired: 1 in, 7 out]
            n296 = call <resource>:"Reset layer template selection.vi"("error in (no error)"=w655, "Data in"=w653) -> ("error out"=w660:errorcluster, "Data out"=w652:T28)  [unwired: 1 in, 7 out]
          }
          event Mouse Down {
            n297 = event-data() -> ()  [unwired: 2 out]
            n298 = call <resource>:"Finalize Text.vi"("error in (no error)"=w681, "Data in"=w680) -> ("error out"=w682:errorcluster, "Data out"=w679:T28)  [unwired: 8 out]
            n299 = call <resource>:"Finalize Movement.vi"("error in (no error)"=w682, "Data in"=w679) -> ("error out"=w678:errorcluster, "Data out"=w676:T28)  [unwired: 1 in, 7 out]
            n300 = call <resource>:"Escape.vi"("error in"=w678, "Data in"=w676) -> ("error out"=w677:errorcluster, "Data out"=w675:T28)  [unwired: 1 in, 7 out]
          }
          event Mouse Down {
            n301 = event-data() -> ("Button"=w686:u16)  [unwired: 1 out]
            n302 = case shown="1" w686 {
              tunnel: w688 -> [w690 w694]
              tunnel: [w690 w693] -> w687
              tunnel: w685 -> [w689 w692]
              tunnel: [w689 w691] -> w684
              frame 0, Default {
              }
              frame 1 {
                # "Left click"
                n303 = call <resource>:"Reset layer template selection.vi"("error in (no error)"=w694, "Data in"=w692) -> ("error out"=w693:errorcluster, "Data out"=w691:T28)  [unwired: 1 in, 7 out]
              }
            }
          }
          event "Preview", "Preview2", "Terminals": Mouse Leave {
            n304 = event-data() -> ()  [unwired: 2 out]
            n305 = Bundle By Name(cluster=w695, "Support.Mouse inside icon?"=FALSE) -> (w697:T28)
          }
          event Mouse Down {
            n306 = event-data() -> ("CtlRef"=w703:refnum<vi>)  [unwired: 1 out]
            n307 = property class="CmbBox (strict)"(reference=w703, error in=w702, "Text.Selection Start"=u32 0 ("Text.Selection:Start"), "Text.Selection End"=u32 1000 ("Text.Selection:End")) -> (error out=w701:errorcluster)  [unwired: 1 out]
          }
          event Value Change {
            n308 = event-data() -> ()  [unwired: 2 out]
            n309 = control-ref of="This VI"() -> (w715:refnum<vi>)
            n310 = call <resource>:"Defer_FP_Updates.vi"("Defer Panel Updates"=TRUE, "error in (no error)"=w714, "lv_icon.vi in"=w715) -> ("error out"=w712:errorcluster, "lv icon.vi out"=w711:refnum<vi>)  [unwired: 7 out]
            n311 = call <resource>:"Add new Layer.vi"("error in"=w712, "Data in"=w716) -> ("error out"=w707:errorcluster, "Data out"=w709:T28)  [unwired: 8 out]
            n312 = call <resource>:"ViewLayer.vi"("Add to Undo?"=TRUE, "error in (no error)"=w707, "Data in"=w709) -> ("error out"=w706:errorcluster, "Data out"=w708:T28)  [unwired: 1 in, 6 out]
            n313 = call <resource>:"Defer_FP_Updates.vi"("error in (no error)"=w706, "lv_icon.vi in"=w711) -> ("error out"=w710:errorcluster)  [unwired: 1 in, 8 out]
          }
          event Value Change {
            n314 = event-data() -> ()  [unwired: 2 out]
            n315 = control-ref of="This VI"() -> (w727:refnum<vi>)
            n316 = Unbundle By Name(w733) -> ("Class.Icon"=w732:refnum<class "Icon.lvclass">)
            n317 = call <resource>:"Defer_FP_Updates.vi"("Defer Panel Updates"=TRUE, "error in (no error)"=w726, "lv_icon.vi in"=w727) -> ("error out"=w725:errorcluster, "lv icon.vi out"=w724:refnum<vi>)  [unwired: 7 out]
            n318 = call-dynamic "GET_All User Layers.vi"("error in (no error)"=w725, "Icon.lvclass in"=w732) -> ("error out"=w739:errorcluster, "User Layer"=w735:refnum<class "Layer.lvclass">[], "Icon.lvclass out"=w734:refnum<class "Icon.lvclass">)  [unwired: 7 out]
            n319 = call <resource>:"Delete Selected Layers.vi"("error in"=w739, "All Layers in"=w735, "Data in"=w733) -> ("error out"=w738:errorcluster, "All Layers out"=w736:refnum<class "Layer.lvclass">[], "Data out"=w730:T28)
            n320 = call-dynamic "SET_UserLayers.vi"("error in (no error)"=w738, "Layers"=w736, "Icon.lvclass in"=w734) -> ("error out"=w737:errorcluster, "Icon.lvclass out"=w731:refnum<class "Icon.lvclass">)  [unwired: 7 in]
            n321 = Bundle By Name(cluster=w730, "Class.Icon"=w731) -> (w729:T28)
            n322 = call <resource>:"Reset layer template selection.vi"("error in (no error)"=w737, "Data in"=w729) -> ("error out"=w718:errorcluster, "Data out"=w720:T28)  [unwired: 1 in, 7 out]
            n323 = call <resource>:"ViewLayer.vi"("Add to Undo?"=TRUE, "error in (no error)"=w718, "Data in"=w720) -> ("error out"=w717:errorcluster, "Data out"=w719:T28)  [unwired: 2 in, 5 out]
            n324 = call <resource>:"Defer_FP_Updates.vi"("error in (no error)"=w717, "lv_icon.vi in"=w724) -> ("error out"=w723:errorcluster)  [unwired: 1 in, 8 out]
          }
          event Panel Close? {
            w741 = FALSE ("Yes")
            n325 = event-data() -> ()  [unwired: 2 out]
            n326 = event-data("Discard?"=TRUE) -> ()  [unwired: 1 in, 1 out]
          }
          event Mouse Up {
            n327 = event-data() -> ()  [unwired: 2 out]
            n328 = Unbundle By Name(w752) -> ("Support.Action"=w750:T32, "Support.Mouse inside icon?"=w755:bool, "Support.Mouse Move Coords"=w751:T31)
            n329 = case shown="False" w755 {
              tunnel: w753 -> [w759 w770]
              tunnel: [w757 w770] -> w748
              tunnel: [w760 w769] -> w746
              tunnel: w752 -> [w761 w769]
              tunnel: w751 -> [w758 _]
              tunnel: w750 -> [w756 _]
              frame False {
                n330 = case shown="\"Move Selection\", \"Tool\"" w756 {
                  tunnel: w761 -> [w763 w768]
                  tunnel: [w763 w767] -> w760
                  tunnel: w759 -> [w762 w766]
                  tunnel: w758 -> [_ w765]
                  tunnel: [w762 w764] -> w757
                  frame "Default", Default {
                  }
                  frame "Move Selection", "Tool" {
                    n331 = call <resource>:"PictureControl_MouseUp.vi"("error in"=w766, "Coords"=w765, "Data in"=w768) -> ("error out"=w764:errorcluster, "Data out"=w767:T28)  [unwired: 4 in, 3 out]
                  }
                }
              }
              frame True {
              }
            }
            n332 = call <resource>:"Add Data to History.vi"("Check special fields? (F)"=TRUE, "Add to Undo?"=TRUE, "error in"=w748, "Data in"=w746) -> ("error out"=w747:errorcluster, "Data out"=w745:T28)  [unwired: 6 out]
          }
          event "Glyphs []": Mouse Down {
            n333 = event-data() -> ("Button"=w779:u16, "Mods.Double Click"=w780:bool, "CtlRef"=w782:refnum<vi>, "Coords"=w783:T31)  [unwired: 1 out]
            n334 = case shown="1" w779 {
              tunnel: w783 -> [_ w792]
              tunnel: w782 -> [_ w791]
              tunnel: [w785 w790] -> w776
              tunnel: w781 -> [w785 w789]
              tunnel: w780 -> [_ w788]
              tunnel: w774 -> [w784 w787]
              tunnel: [w784 w786] -> w772
              frame 0, Default {
              }
              frame 1 {
                # "Left click"
                n335 = call <resource>:"Mouse Down_Glyphs.vi"("Double Click"=w788, "Coords"=w792, "error in"=w789, "CtlRef"=w791, "Data in"=w787) -> ("error out"=w790:errorcluster, "Data out"=w786:T28)  [unwired: 1 in, 4 out]
              }
            }
            n336 = call <resource>:"Reset layer template selection.vi"("error in (no error)"=w776, "Data in"=w772) -> ("error out"=w775:errorcluster, "Data out"=w773:T28)  [unwired: 1 in, 7 out]
            n337 = call <resource>:"Update glyph path string.vi"("error in (no error)"=w775, "Data in"=w773) -> ("error out"=w777:errorcluster, "Data out"=w771:T28)  [unwired: 1 in, 7 out]
          }
          event Mouse Down {
            n338 = event-data() -> ()  [unwired: 2 out]
            n339 = call <resource>:"Escape.vi"("error in"=w794, "Data in"=w796) -> ("error out"=w793:errorcluster, "Data out"=w795:T28)  [unwired: 1 in, 7 out]
          }
          event "Glyphs", "Templates": Item Close; "Glyphs", "Templates": event #0x1e {
            n340 = event-data() -> ("CtlRef"=w797:refnum<vi>)  [unwired: 1 out]
            n341 = call <resource>:"DealWithScrollbars.vi"("error in (no error)"=w799, "Tree"=w797) -> ("error out"=w798:errorcluster)  [unwired: 9 in]
          }
          event Value Change {
            n342 = event-data() -> ()  [unwired: 2 out]
            n343 = Unbundle By Name(w803) -> ("Ref.GlyphLoadAnimation"=w801:refnum<vi>, "Ref.refreshGlyphs"=w802:refnum<vi>)
            n344 = call <resource>:"Launch Dynamically Load Graphics.vi"("User events"=w804, "Path"=Pathes."Glyphs", "error in (no error)"=w806, "button ref"=w802, "animatedDecoration ref"=w801) -> ("error out"=w805:errorcluster)  [unwired: 1 in, 5 out]
          }
          event Value Change {
            n345 = event-data() -> ()  [unwired: 2 out]
            n346 = Unbundle By Name(w810) -> ("Ref.TemplateLoadAnimation"=w808:refnum<vi>, "Ref.refreshTemplates"=w809:refnum<vi>)
            n347 = call <resource>:"Launch Dynamically Load Graphics.vi"("User events"=w811, "Path"=Pathes."Icon Templates", "error in (no error)"=w813, "button ref"=w809, "animatedDecoration ref"=w808) -> ("error out"=w812:errorcluster)  [unwired: 1 in, 5 out]
          }
        }
        n348 = case shown="True" w151 {
          tunnel: [_ w166] -> w155
          tunnel: w154 -> [w163 w169]
          tunnel: [w163 w168] -> w153
          tunnel: "Tools" -> [_ w167]
          tunnel: w147 -> [w162 w165]
          tunnel: [w162 w164] -> w146
          frame False {
          }
          frame True {
            n349 = call <resource>:"DrawIcon.vi"("Tools"=w167, "error in (no error)"=w169, "Data in"=w165) -> ("error out"=w168:errorcluster, "Icon"=w166:picture, "Data out"=w164:T28, "RGB"=→"RGB":string, "XYL"=→"XYZ":string)  [unwired: 2 in, 2 out]
            "Icon" <- w166
            "Preview" <- w166
          }
        }
        n350 = Unbundle By Name(w154) -> ("status"=w160:bool)
        n351 = Or(x=w160, y=w159) -> (x .or. y?=w158:bool)
      }
      n352 = call <resource>:"Buffer for lossless tracking.vi"("Ref Cluster"=w128, "User events"=w131, "error in (no error)"=w133, "Buffer"=w132) -> ()  [unwired: 8 out]
      n353 = call <resource>:"Extract LV Icon Data.vi"("error in (no error)"=w122, "LabVIEW Icon in (original)"=w120, "Data in"=w124) -> ("error out"=w121:errorcluster, "LabVIEW Icon out"=w123:string, "Data out"=w119:T28)  [unwired: 6 in]
      n354 = call <vilib>:"Get Image Data.vi"("Pic In"=w140) -> ("image data out"=w127:T4)  [unwired: 2 in, 8 out]
      n355 = call <vilib>:"Get Image Data.vi"("depth (24)"=1 ("depth"), "Pic In"=w140) -> ("image data out"=w138:T4)  [unwired: 2 in, 7 out]
      n356 = call <resource>:"SetCursor.vi"("Radio Buttons"=Tools."Select", "Data in"=w119) -> ("Data out"=w118:T28)  [unwired: 8 in, 1 out]
      n357 = Unbundle By Name(w121) -> ("code"=w141:i32)
      n358 = flat-sequence {
        tunnel: w144 -> [w829]
        tunnel: w142 -> [w826]
        tunnel: w121 -> [w825]
        tunnel: w131 -> [w823]
        tunnel: w118 -> [w819]
        tunnel: w115 -> [w817]
        tunnel: [w817] -> w114
        tunnel: [w816] -> w113
        tunnel: [w815] -> w112
        tunnel: w111 -> [w815]
        tunnel: w114 -> [w834]
        tunnel: w113 -> [w833]
        tunnel: w112 -> [w831]
        frame #0 {
          n359 = Unbundle By Name(w823) -> ("Global stop?"=w822:refnum<user-event>, "Templates"=w821:refnum<user-event>, "Glyphs"=w820:refnum<user-event>)
          n360 = Unbundle(w829) -> ("Events"=w828:refnum<event-registration>)
          n361 = call <resource>:"Write INI Tokens and VI Tags.vi"("error in (no error)"=w825, "Data in"=w819) -> ("error out"=w818:errorcluster)  [unwired: 1 in, 8 out]
          n362 = Unregister For Events(event registration refnum=w828) -> ()  [unwired: 1 in, 1 out]
          n363 = flat-sequence {
            tunnel: w818 -> [_]
            tunnel: [w830] -> w816
            frame #0 {
              n364 = call <resource>:"Call Keep IE in Memory.vi"() -> ()  [unwired: 1 out]
            }
            frame #1 {
              n365 = property class="VI"() -> ("Front Panel.WinBounds"=w830:T37)  [unwired: 2 in, 2 out]
            }
          }
          n366 = Release Notifier(notifier=w826, force destroy? (F)=TRUE) -> ()  [unwired: 1 in, 3 out]
          n367 = Generate User Event(user event=w822, event data cluster=TRUE) -> ()  [unwired: 2 in, 2 out]
          n368 = Destroy User Event(user event=w821) -> ()  [unwired: 1 in, 1 out]
          n369 = Destroy User Event(user event=w820) -> ()  [unwired: 1 in, 1 out]
        }
        frame #1 {
          n370 = Equal?(x=w833, y=w834) -> (x = y?=w832:bool)
          n371 = case shown="False" w832 {
            tunnel: w833 -> [w842 _]
            tunnel: w831 -> [w835 _]
            frame False {
              # "Bounds changed...write new bounds\nto INI file"
              n372 = Unbundle(w842) -> ("Left"=w841:i16, "Top"=w840:i16, "Right"=w839:i16, "Bottom"=w838:i16)
              n373 = Format Into String(format string="%d,%d,%d,%d", w841, w840, w839, w838) -> (resulting string=w836:string)  [unwired: 2 in, 1 out]
              n374 = call-by-ref "?"("value"=w836, "key"=w835) -> ()  [unwired: 3 in, 7 out]
            }
            frame True {
              # "Bounds didn't change while window was\nopen...don't do anything"
            }
          }
        }
        frame #2 {
          n375 = invoke class="VI" method="FP.Close"() -> ()  [unwired: 3 in, 3 out]
        }
      }
      n376 = call-dynamic "GET_Notifier.vi"("error in (no error)"=w125, "Ants.lvclass in"=w129) -> ("error out"=w136:errorcluster, "Notifier"=w142:refnum<notifier>, "Ants.lvclass out"=w137:refnum<class "Ants.lvclass">)  [unwired: 7 out]
      n377 = call <resource>:"RunningAnts.vi"("error in (no error)"=w136, "Ants in"=w137) -> ()  [unwired: 10 out]
    }
    frame Error {
      n378 = Unbundle By Name(w844) -> ("code"=w845:i32)
      n379 = call <vilib>:"Simple Error Handler.vi"("error in (no error)"=w844) -> ()  [unwired: 4 in, 5 out]
    }
  }
  "BW icon out" <- w56
  "Error code out" <- w61
  "Color icon out" <- w37
  "LabVIEW Icon out" <- w30
